vi "多点监测上位机-服务器版.vi"() -> ()   [LabVIEW 2013]
uses:
  <vilib>/Utility/miscctls.llb/LVRowAndColumnTypeDef.ctl
  <vilib>/Utility/miscctls.llb/LVRowAndColumnUnsignedTypeDef.ctl
  <vilib>/Platform/TimedLoop/XDataNode/timing_clust.ctl
  <vilib>/Platform/TimedLoop/XDataNode/nitl_modes.ctl
  <vilib>/Platform/TimedLoop/XDataNode/wakeup.ctl
  <vilib>/Utility/xml.llb/Read From XML File(string).vi
  <vilib>/sound2/lvsound2.llb/Sound File Info (path).vi
  <vilib>/sound2/lvsound2.llb/Sound File Read Open.vi
  <vilib>/sound2/lvsound2.llb/Sound File Read (DBL).vi
  <vilib>/Utility/file.llb/Read From Spreadsheet File (string).vi
  <vilib>/Utility/xml.llb/Write to XML File(string).vi
  <vilib>/Utility/file.llb/Write To Spreadsheet File (string).vi
  <vilib>/Utility/inputDevices.llb/closeMouse.vi
  <vilib>/Utility/inputDevices.llb/mouseAcquire.vi
  <vilib>/Platform/TimedLoop/XDataNode/XDataNode.xnode
  <vilib>/Platform/TimedLoop/XDataNode/XDNodeRunTimeDep.lvlib
panel:
  out "监-停止信号":refnum<vi>
  out "监测数量限值":cluster{"min":i32, "max":i32}
  in  "报警列表提示":string[](array[string])=["选行技巧：按住 ctl 可离散选择，按住 shift 可范围选择，ctl+A 选择全部行", "右键菜单：多选后 某些项可批量操作", "双击“状态”列：启用或禁用设备（某些版本中禁用此功能）", "双击“设备信息”列：修改设备信息", "双击“一级限值”列：修改报警限值", "双击“网络地址”列：删除设备", "双击“空白行”：添加设备"]
  in  "设备列表提示":string[](array[string])=["选行技巧：按住 ctl 可离散选择，按住 shift 可范围选择，ctl+A 选择全部行", "右键菜单：多选后 某些项可批量操作", "双击“状态”列：启用或禁用设备（某些版本中禁用此功能）", "双击“设备信息”列：修改设备信息", "双击“一级限值”列：修改报警限值", "双击“网络地址”列：删除设备", "双击“空白行”：添加设备"]
  in  "停止信号":enum16{"内部停止信号", "外部停止信号"}(ring)
  out "数组":errorcluster[](array[cluster])
  out "在线探头索引映射":i32[](array[numeric])
  out "在线探头":T1(array[cluster])
  out "连接断开-事件":refnum<user-event>
  out "新连接-事件":refnum<user-event>
  out "新纪录通知VI":refnum<vi>
  in  "新记录簇":cluster{"新记录列表行":string[], "对应缓存文件":string}[](array[cluster])
  in  "报警记录数":i32
  out "蜂鸣音效":waveform(dbl)[](array[waveform]) caption="数据"
  in  "新记录？":bool=TRUE
  in  "Right":i16
  in  "Left":i16
  out "最终事件":i32
  in  "所有探头数":i32
  out "定时循环结构名称":string="采集探头属性"
  in  "测量状态":enum16{"正常", "一级报警", "二级报警"}(ring)
  in  "通信单元-探头属性引用[]":refnum<vi>[](array[refnum])
  in  "通信分支-改动项引用[]":refnum<vi>[](array[refnum])
  in  "探头属性数组":T1(array[cluster])
  in  "菜单项-报警列表":enum16{"刷新", "预览并生成报表", "删除记录", "复制选中项至剪贴板"}(ring)=enum."预览并生成报表"
  in  "菜单项-实时列表":T2(ring)=enum."禁用"
  out "监测窗口VI":refnum<vi>
  out "报警记录缓存数据文件":string[](array[string])
  in  "状态与编辑":bool
  in  "监测模式":bool caption="方格样式"
  in  "查看报表":bool caption="方格样式"
  in  "设置":bool
  in  "通知设置":bool caption="方格样式"
  in  "帮助":bool
  out "公司LOGO与型号":bool
  out "设备列表标题":enum16{"设备管理列表"}(ring)
  out "设备列表操作提示":string
  in  "状态栏-项名[]":string[](array[string])
  in  "通信分支-VI引用[]":refnum<vi>[](array[refnum])
  in  "实时数据列表":i32[](listbox)
  out "报警列表标题":enum16{"报警记录列表"}(ring)
  out "报警列表操作提示":string
  in  "T:G,F:B":bool
  in  "回复背景色锁":bool
  in  "等待时间（毫秒）":u32=10
  in  "报警记录列表":i32[](listbox)
  in  "状态类型":enum16{"全部", "报警", "通信", "设置"}(ring)
  in  "暂停更新？":bool
  in  "状态栏":i32(listbox)
  in  "开机启动":bool
  in  "device ID":refnum<k1> caption="设备ID"
  in  "监测模式？":bool
  out "点到行列-实时列表":T3 caption="单元格位置"
  out "点到行列-报警记录":T3 caption="单元格位置"
  out "停止":bool=TRUE
  in  "清除状态":bool
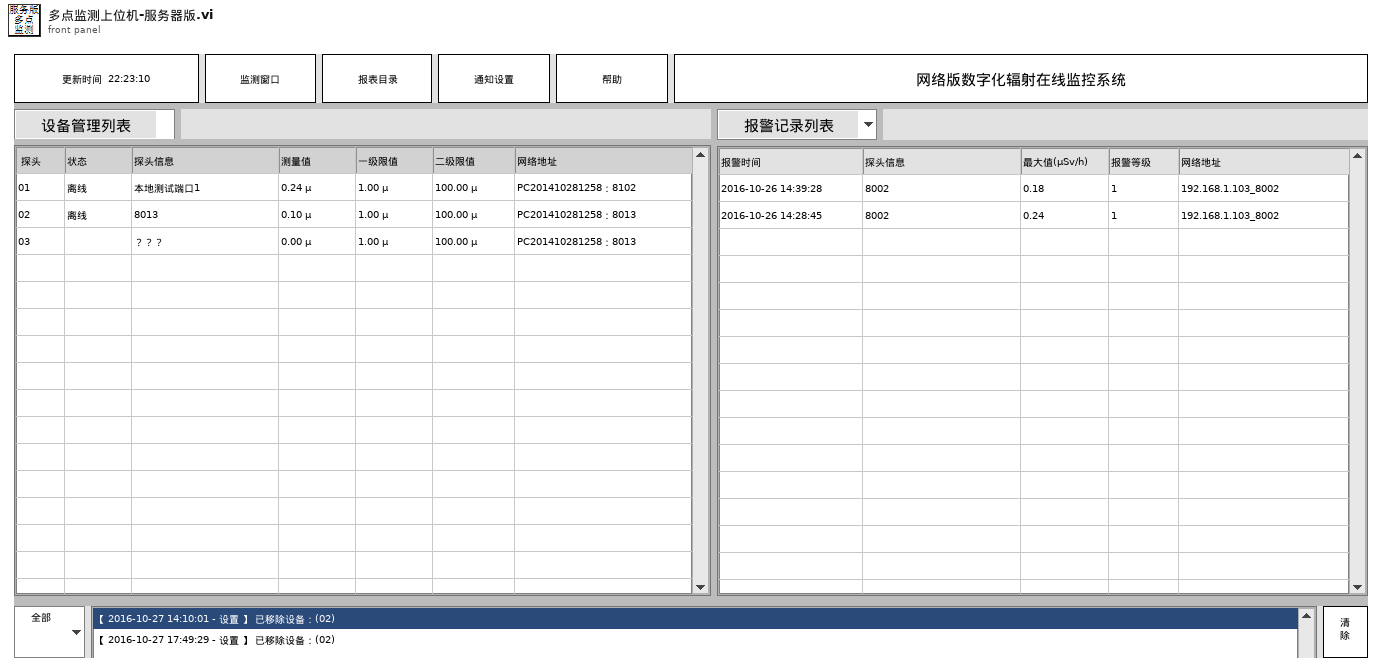
[diagram p1: front panel]
types:
  T1 = cluster{"探头地址与信息":cluster{"网络地址":cluster{"IP":string, "port":u16}, "探头信息":string}, "测量值":cluster{"时间":timestamp, "数值":dbl}, "限值":cluster{"限值1":dbl, "限值2":dbl}, "探头状态":enum16{"正常", "离线", "禁用", "一级报警", "二级报警"}}[]
  T2 = enum16{"启用", "禁用", "修改探头信息", "修改报警限值", "设备排序", "添加设备", "删除设备"}
  T3 = typedef "LVRowAndColumnTypeDef.ctl" = cluster{"Row":i32, "Column":i32}
  T4 = typedef "LVRowAndColumnUnsignedTypeDef.ctl" = cluster{"Row":u32, "Column":u32}
  T5 = enum32{"Invalid", "Standard", "Closed", "Hidden", "Minimized", "Maximized"}
  T6 = enum8{"Enabled", "Disabled", "Disabled and Grayed Out"}
  T7 = typedef "XDNodeRunTimeDep.lvlib/timing_clust.ctl" = cluster{"Expected End [f-1]":u64, "Actual End [f-1]":u64, "Finished Late? [f-1]":bool, "Expected End [i-1]":u64, "Actual End [i-1]":u64, "Finished Late? [i-1]":bool, "Expected Start [i]":u64, "Actual Start [i]":u64, "Expected Start [f]":u64, "Actual Start [f]":u64, "Source Name":string, "Structure Name":string, "Period":i64, "Deadline":i64, "Offset":i64, "Start":i64, "Priority":i32, "Timeout":i32, "Mode":T8, "Wakeup Reason":T9, "Error":errorcluster, "Source Type":string, "Secondary Source Type":string, "Global End Time":u64, "Global Start Time":u64, "Frame Duration":u64, "Iteration Duration":u64, "Assigned CPU":i32, "I/O Scan Engine Mode":u32}
  T8 = typedef "XDNodeRunTimeDep.lvlib/nitl_modes.ctl" = enum32{"No Change", "Process missed periods, maintain original phase", "Discard missed periods, maintain original phase", "Process missed periods, ignore original phase", "Discard missed periods, ignore original phase"}
  T9 = typedef "XDNodeRunTimeDep.lvlib/wakeup.ctl" = enum32{"Normal", "Aborted", "Asynchronous wakeup", "Timing source error", "Timed loop error", "Timeout"}
  T10 = cluster{"企业编号":string, "员工编号":string, "通道号":string, "密码":string, "联系人数组":cluster{"姓名":string, "手机号":string}[]}
  T11 = cluster{"连接ID":refnum<k5>, "IP地址":string, "端口":u16}
  T12 = typedef "Sound File Refnum.ctl" = refnum<file>
  T13 = typedef "LVRectTypeDef.ctl" = cluster{"Left":i16, "Top":i16, "Right":i16, "Bottom":i16}
  T14 = cluster{"探头地址与信息":cluster{"网络地址":cluster{"IP":string, "port":u16}, "探头信息":string}, "测量值":cluster{"时间":timestamp, "数值":dbl}, "限值":cluster{"限值1":dbl, "限值2":dbl}, "探头状态":enum16{"正常", "离线", "禁用", "一级报警", "二级报警"}}
  T15 = typedef "LVPoint32TypeDef.ctl" = cluster{"Horizontal":i32, "Vertical":i32}
  T16 = cluster{"button 1":bool, "button 2":bool, "button 3":bool, "button 4":bool}
  T17 = cluster{"Shift":bool, "Ctrl":bool, "Alt":bool, "Cmd":bool, "Opt":bool}
  T18 = cluster{"探头信息":string, "启用？":bool, "改动项":enum16{"未改动", "改动-探头信息", "改动-启用状态", "改动-限值"}, "限值":cluster{"限值1":dbl, "限值2":dbl}}
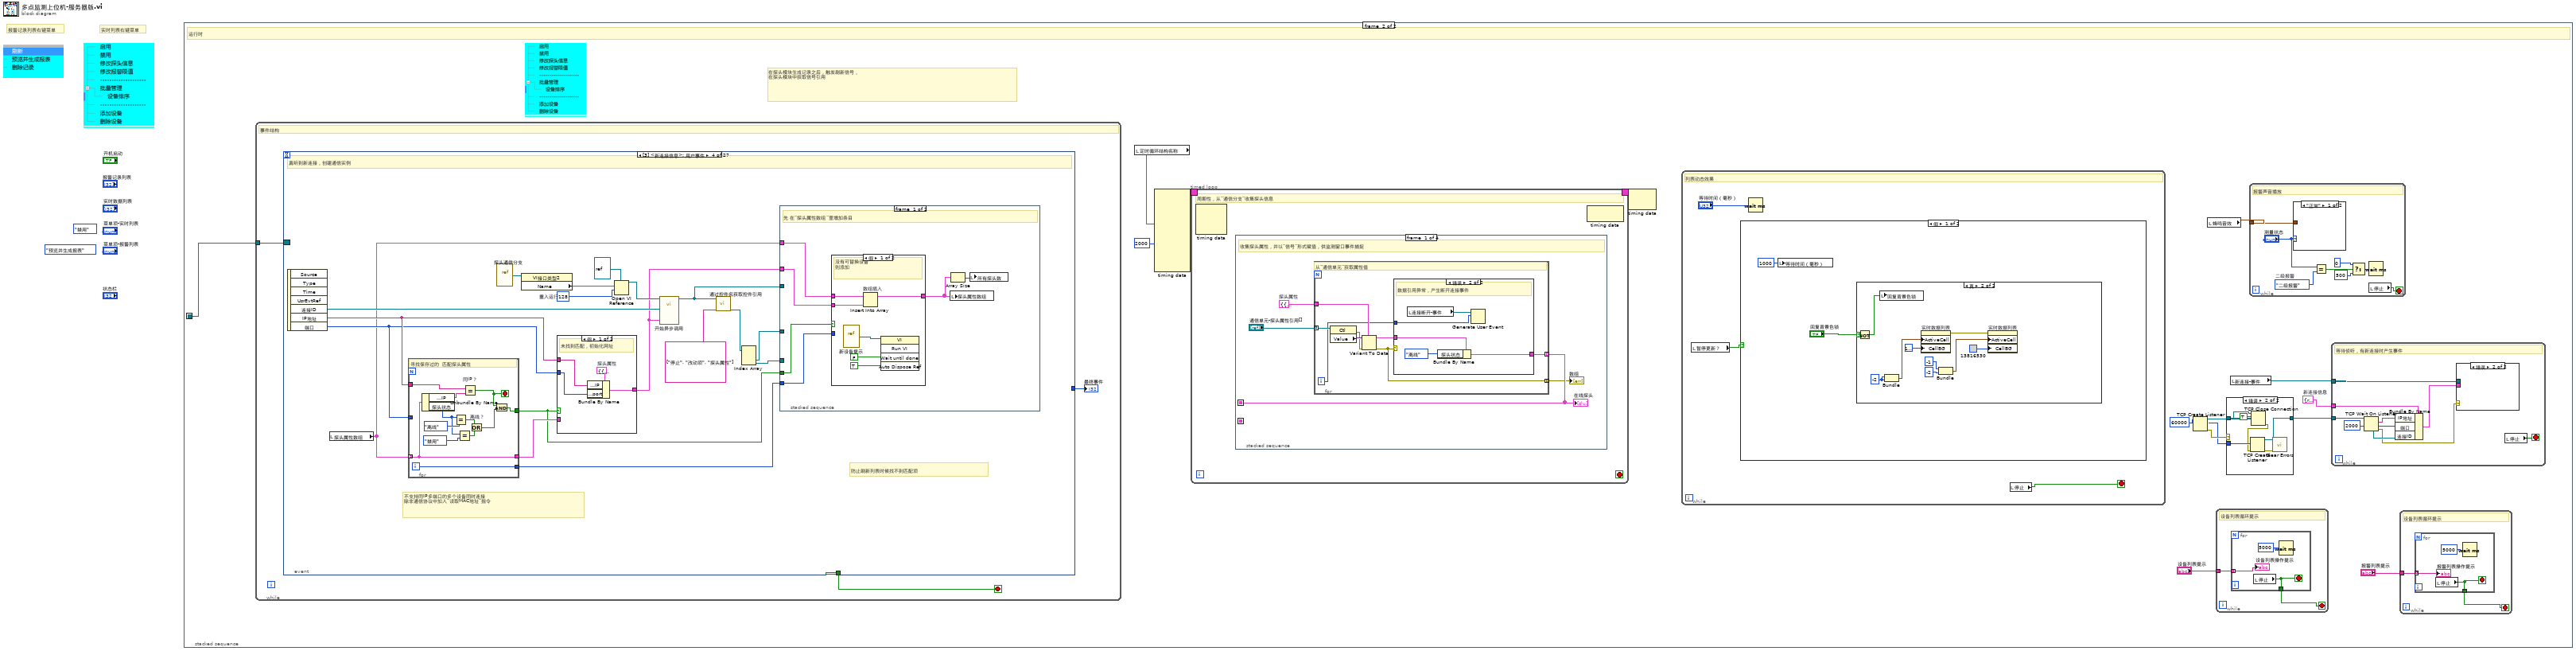
[diagram p0: block diagram]
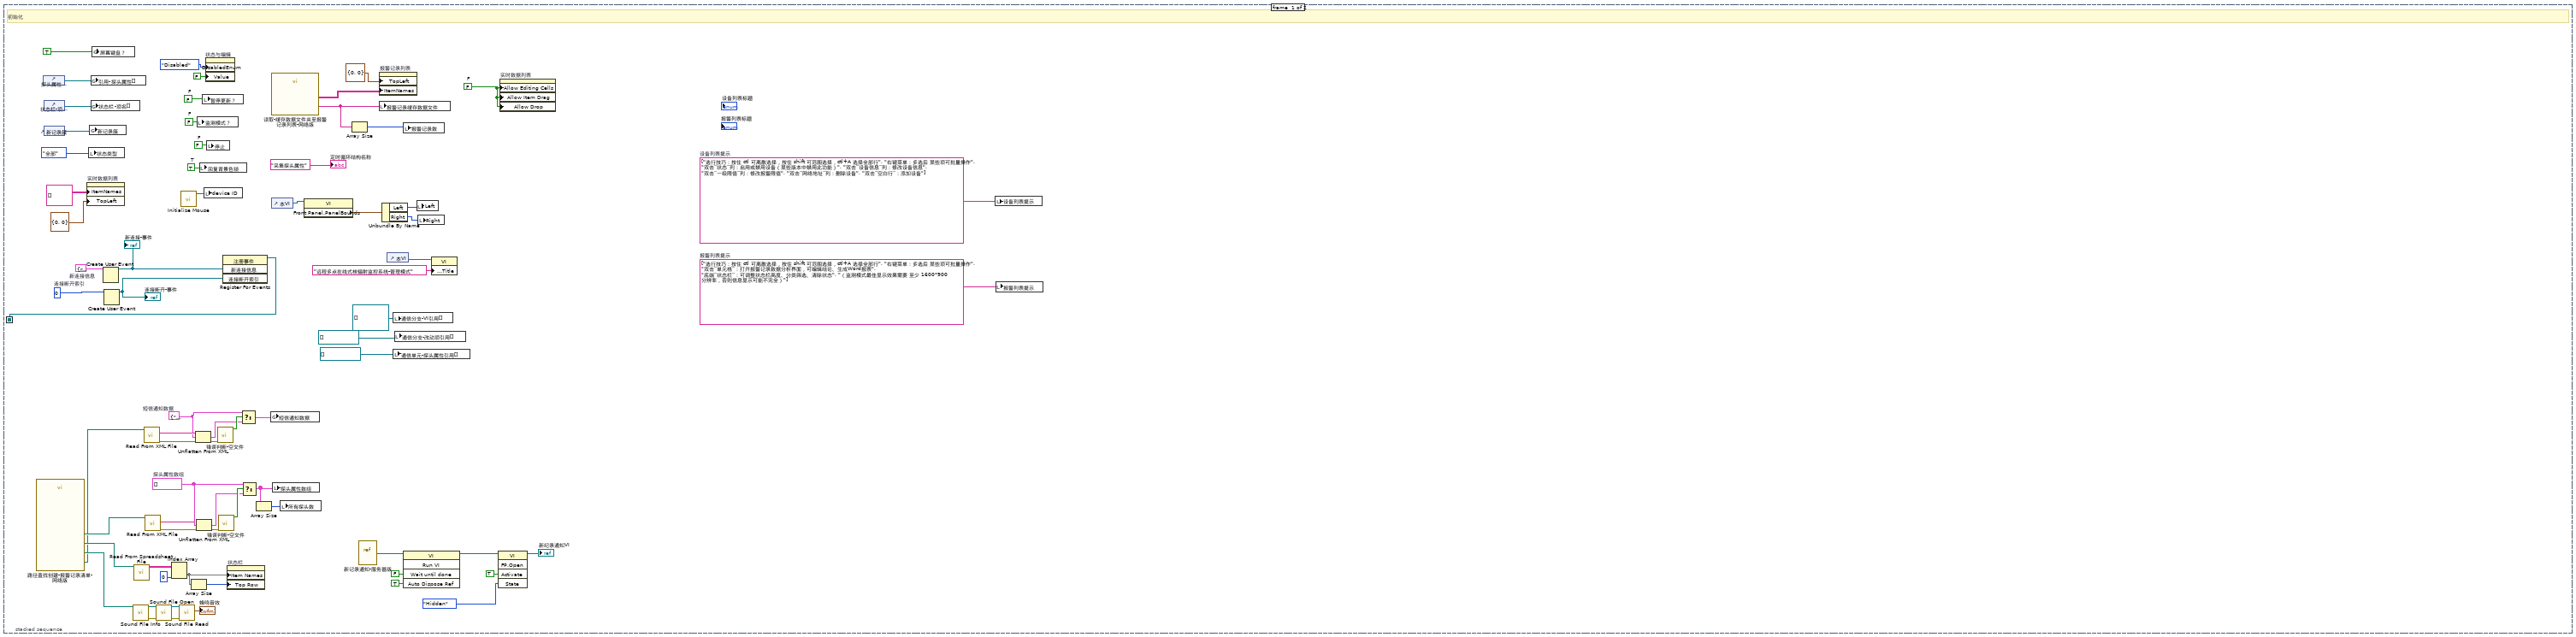
[diagram p2: hidden frame]
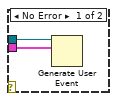
[diagram p4: hidden frame]
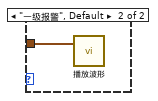
[diagram p5: hidden frame]
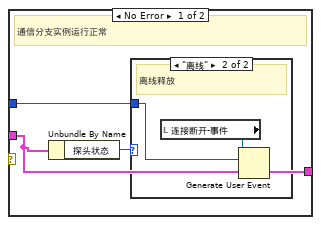
[diagram p6: hidden frame]
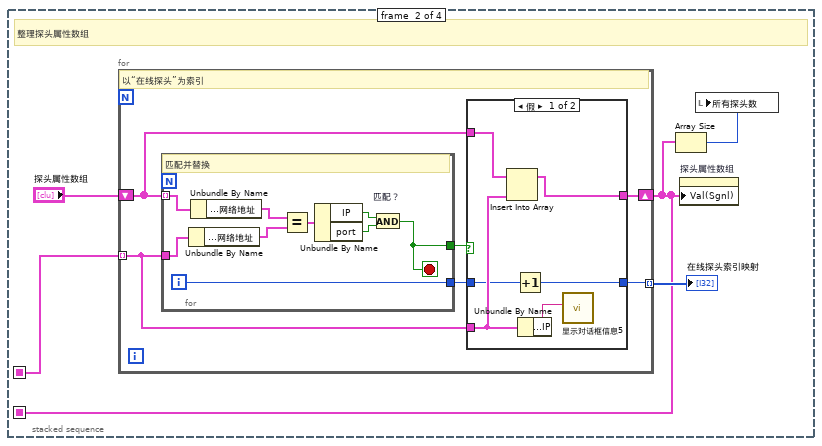
[diagram p8: hidden frame]
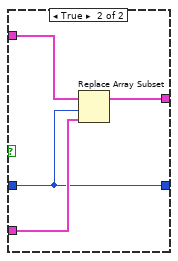
[diagram p9: hidden frame]
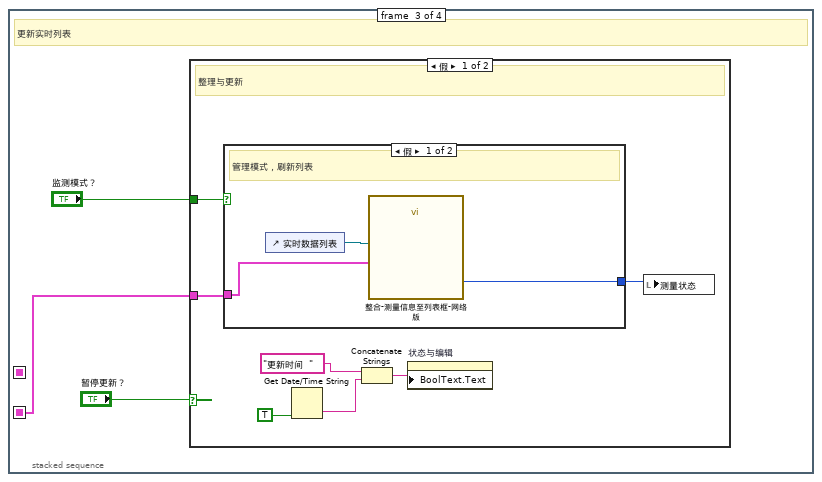
[diagram p10: hidden frame]
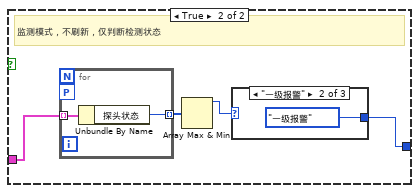
[diagram p11: hidden frame]
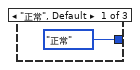
[diagram p12: hidden frame]
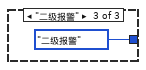
[diagram p13: hidden frame]
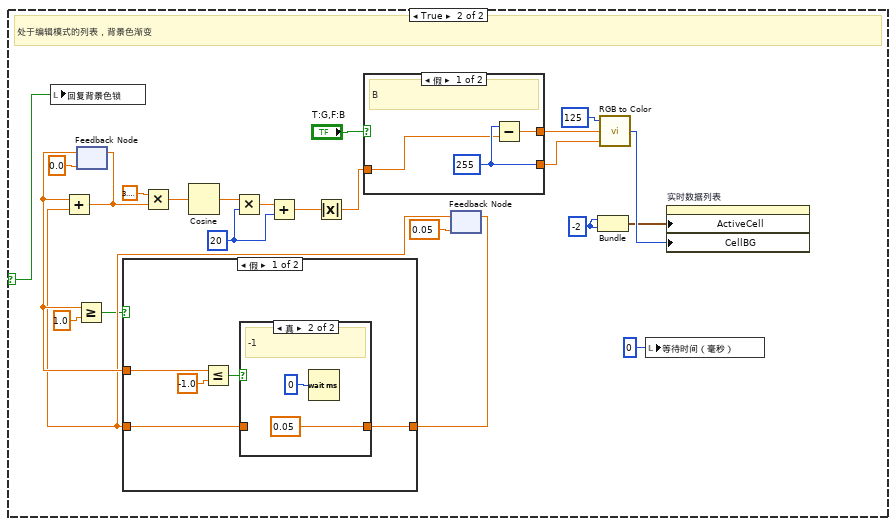
[diagram p17: hidden frame]
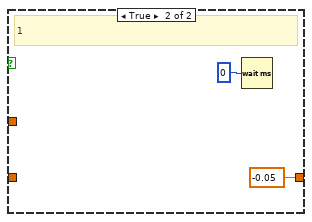
[diagram p19: hidden frame]
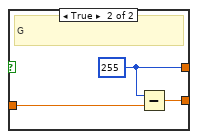
[diagram p20: hidden frame]
diagram:
  (unwired) enum16{"刷新", "预览并生成报表", "删除记录", "复制选中项至剪贴板"}."预览并生成报表" ("菜单项-报警列表")
  (unwired) T2."禁用" ("菜单项-实时列表")
  # "报警记录列表右键菜单"
  # "实时列表右键菜单"
  n1 = stacked-sequence {
    seq-local: [w24 _] -> [_ w82]
    frame #0 {
      w7 = string[] ["选行技巧：按住 ctl 可离散选择，按住 shift 可范围选择，ctl+A 选择全部行", "右键菜单：多选后 某些项可批量操作", "双击“单元格”：打开报警记录数据分析界面，可编辑结论、生成Word报表", "底端“状态栏”：可调整状态栏高度、分类筛选、清除状态", "（监测模式最佳显示效果需要 至少 1600*900 分辨率，否则信息显示可能不完全）"]  # 报警列表提示
      w6 = string[] ["选行技巧：按住 ctl 可离散选择，按住 shift 可范围选择，ctl+A 选择全部行", "右键菜单：多选后 某些项可批量操作", "双击“状态”列：启用或禁用设备（某些版本中禁用此功能）", "双击“设备信息”列：修改设备信息", "双击“一级限值”列：修改报警限值", "双击“网络地址”列：删除设备", "双击“空白行”：添加设备"]  # 设备列表提示
      w10 = T10 {"企业编号"="", "员工编号"="", "通道号"="", "密码"="", "联系人数组"=[]}  # 短信通知数据
      w22 = 0  # 连接断开索引
      w26 = T11 {"连接ID"=refnum, "IP地址"="", "端口"=0}  # 新连接信息
      w50 = TRUE  # T
      w51 = FALSE  # F
      w59 = T1 []  # 探头属性数组
      w68 = FALSE  # F
      w64 = FALSE  # F
      w71 = FALSE  # F
      # "初始化"
      n2 = call "路径查找创建-报警记录清单-网络版.vi"() -> ("探头属性配置文件"=w58:path, "状态栏信息文件"=w54:path, "蜂鸣音效文件路径"=w38:path, "短信通知配置文件"=w13:path)  [unwired: 1 in, 7 out]
      n3 = control-ref of="探头属性数组"() -> (w62:refnum<vi>)
      n4 = control-ref of="状态栏-项名[]"() -> (w70:refnum<vi>)
      n5 = control-ref of="新记录簇"() -> (w35:refnum<vi>)
      n6 = property on="实时数据列表" class="MCListbox (严格)"("ItemNames"=string[][] [] ("项名"), "TopLeft"=T4 {"Row"=0, "Column"=0} ("左上可见单元格")) -> ()  [unwired: 2 in, 2 out]
      n7 = local write "状态类型"(enum16{"全部", "报警", "通信", "设置"}."全部" ("状态类型")) -> ()
      n8 = global write "全局变量-35点监测.vi" "新记录簇"(w35) -> ()
      n9 = global write "全局变量-35点监测.vi" "引用-探头属性[]"(w62) -> ()
      n10 = global write "全局变量-35点监测.vi" "状态栏-项名[]"(w70) -> ()
      n11 = global write "全局变量-35点监测.vi" "屏幕键盘？"(TRUE ("屏幕键盘？")) -> ()
      n12 = Create User Event(user event datatype=w26) -> (user event=w25:refnum<user-event>)  [unwired: 1 in, 1 out]
      "新连接-事件" <- w25
      n13 = Create User Event(user event datatype=w22) -> (user event=w23:refnum<user-event>)  [unwired: 1 in, 1 out]
      "连接断开-事件" <- w23
      n14 = call-poly <vilib>:"Sound File Info.vi"("path"=w38) -> ("error out"=w40:errorcluster, "path out"=w41:path)  [unwired: 7 in, 2 out]
      n15 = call-poly <vilib>:"Read From Spreadsheet File.vi"("file path (dialog if empty)"=w54) -> ("all rows"=w53:string[][])  [unwired: 6 in, 4 out]
      n16 = call-poly <vilib>:"Read From XML File.vi"("XML File Path"=w13) -> ("error out"=w15:errorcluster, "XML Elements"=w12:string)  [unwired: 8 in, 1 out]
      n17 = call-poly <vilib>:"Read From XML File.vi"("XML File Path"=w58) -> ("error out"=w56:errorcluster, "XML Elements"=w55:string)  [unwired: 8 in, 1 out]
      n18 = call-poly <vilib>:"Sound File Open.vi"("error in (no error)"=w40, "path"=w41) -> ("error out"=w39:errorcluster, "sound file refnum"=w42:T12)  [unwired: 8 in]
      n19 = Index Array(array=w53, index (col)=0 ("禁用的索引 (列)")) -> (element=w19:string[])  [unwired: 1 in]
      n20 = call-poly <vilib>:"Sound File Read.vi"("error in (no error)"=w39, "sound file refnum"=w42) -> ("data"=→"蜂鸣音效":waveform(dbl)[])  [unwired: 5 in, 4 out]
      n21 = call <vilib>:"Initialize Mouse.vi"() -> ("device ID"=w69:refnum<k1>)  [unwired: 10 in, 1 out]
      n22 = Array Size(array=w19) -> (size(s)=w18:i32)
      n23 = Unflatten From XML(xml string=w12, type=w10, error in (no error)=w15) -> (value=w9:T10, error out=w14:errorcluster)
      n24 = Unflatten From XML(xml string=w55, type=w59, error in (no error)=w56) -> (value=w57:T1, error out=w60:errorcluster)
      n25 = local write "监测模式？"(w68) -> ()
      n26 = local write "回复背景色锁"(w50) -> ()
      n27 = local write "暂停更新？"(w51) -> ()
      n28 = local write "device ID"(w69) -> ()
      n29 = property on="状态与编辑" class="Bool (严格)"("DisabledEnum"=T6."Disabled" ("禁用"), "Value"=FALSE ("状态与编辑")) -> ()  [unwired: 2 in, 2 out]
      n30 = local write "停止"(w71) -> ()
      n31 = call "错误判断-空文件.vi"("错误输入"=w14) -> ("空文件？"=w11:bool)  [unwired: 9 in, 1 out]
      n32 = call "错误判断-空文件.vi"("错误输入"=w60) -> ("空文件？"=w61:bool)  [unwired: 9 in, 1 out]
      n33 = register-events(w25, w23) -> (reference out=w24:refnum<event-registration>)  [unwired: 2 in, 1 out]
      n34 = property on="状态栏" class="LstBox (严格)"("Item Names"=w19, "Top Row"=w18) -> ()  [unwired: 2 in, 2 out]
      n35 = Select(t=w10, s=w11, f=w9) -> (s? t:f=w8:T10)
      n36 = Select(t=w59, s=w61, f=w57) -> (s? t:f=w20:T1)
      n37 = Array Size(array=w20) -> (size(s)=w21:i32)
      n38 = global write "全局变量-35点监测.vi" "短信通知数据"(w8) -> ()
      n39 = call "读取-缓存数据文件夹至报警记录列表-网络版.vi"() -> ("文件名"=w37:string[], "报警记录列表"=w45:string[][])  [unwired: 8 in, 2 out]
      n40 = control-ref of="本VI"() -> (w49:refnum<vi>)
      n41 = local write "探头属性数组"(w20) -> ()
      n42 = local write "所有探头数"(w21) -> ()
      n43 = property class="VI"(reference=w49) -> ("Front Panel.PanelBounds"=w48:T13)  [unwired: 1 in, 2 out]
      n44 = Array Size(array=w37) -> (size(s)=w36:i32)
      n45 = vi-ref "新记录通知-服务器版.vi"() -> (w34:refnum<vi>)
      n46 = local write "报警记录缓存数据文件"(w37) -> ()
      n47 = property on="报警记录列表" class="MCListbox (严格)"("TopLeft"=T4 {"Row"=0, "Column"=0} ("左上可见单元格"), "ItemNames"=w45) -> ()  [unwired: 2 in, 2 out]
      n48 = Unbundle By Name(w48) -> ("Left"=w47:i16, "Right"=w46:i16)
      n49 = control-ref of="本VI"() -> (w17:refnum<vi>)
      n50 = local write "通信单元-探头属性引用[]"(refnum<vi>[] [] ("通信单元-探头属性引用[]")) -> ()
      n51 = local write "通信分支-VI引用[]"(refnum<vi>[] [] ("通信分支-VI引用[]")) -> ()
      n52 = local write "通信分支-改动项引用[]"(refnum<vi>[] [] ("通信分支-改动项引用[]")) -> ()
      n53 = local write "报警记录数"(w36) -> ()
      n54 = invoke class="VI" method="Run VI"(reference=w34, "Wait until done"=FALSE ("结束前等待"), "Auto Dispose Ref"=TRUE ("自动销毁引用")) -> (reference out=w31:refnum<vi>)  [unwired: 2 in, 4 out]
      n55 = local write "Left"(w47) -> ()
      n56 = local write "Right"(w46) -> ()
      n57 = property class="VI"(reference=w17, "Front Panel.Title"="远程多点在线式核辐射监控系统-管理模式" ("前面板窗口:标题")) -> ()  [unwired: 1 in, 2 out]
      n58 = invoke class="VI" method="FP.Open"(reference=w31, "Activate"=TRUE ("激活？"), "State"=T5."Hidden" ("状态")) -> (reference out=→"新纪录通知VI":refnum<vi>)  [unwired: 2 in, 4 out]
      n59 = property on="实时数据列表" class="多列列表框 (严格)"("Allow Editing Cells"=w64, "Allow Item Drag"=w64, "Allow Drop"=w64) -> ()  [unwired: 2 in, 2 out]
      n60 = local write "设备列表提示"(w6) -> ()
      n61 = local write "报警列表提示"(w7) -> ()
      "定时循环结构名称" <- "采集探头属性"
    }
    frame #1 {
      w80 = T11 {"连接ID"=refnum, "IP地址"="", "端口"=0}  # 新连接信息
      # "在探头模块生成记录之后，触发刷新信号，\n在探头模块中获取信号引用"
      # "运行时"
      n62 = while {
        tunnel: w82 -> [w261]
        stop <- w263 stop-if-true
        # "事件结构"
        n63 = event shown="[3] <新连接信息>: 用户事件" {
          selector: w261 -> [_ _ _ _ _ _ _ _ _ _ _ _ _ _ _ _ _ _ _ _ _ _ _ _ _ _ _]
          dyn-events: _ -> [_ _ _ _ _ _ _ _ _ _ _ _ _ _ _ _ _ _ _ _ _ _ _ _ _ _ _]
          timeout: _ -> [_ _ _ _ _ _ _ _ _ _ _ _ _ _ _ _ _ _ _ _ _ _ _ _ _ _ _]
          tunnel: [_ w267 _ _ _ _ _ _ _ _ _ _ _ _ _ _ _ _ _ _ _ _ _ _ _ _ _] -> w263
          tunnel: [0 1 _ _ _ 2 3 4 5 6 7 _ 8 9 10 _ _ _ _ _ _ 17 _ _ _ _ _] -> w262
          event Timeout {
            # "超时刷新历史记录"
            n64 = event-data() -> ()  [unwired: 1 in, 3 out]
          }
          event "停止信号": Value Change {
            # "触发停止，关闭通信单元，关闭TCP连接"
            n65 = event-data() -> ("NewVal"=w265:enum16{"内部停止信号", "外部停止信号"})  [unwired: 1 in, 5 out]
            n66 = case shown="\"内部停止信号\", 默认" w265 {
              tunnel: [w268 w269] -> w267
              frame "内部停止信号", Default {
                # "内部停止信号，有弹窗"
                n67 = call "显示对话框信息3"() -> ("确定"=w268:bool)  [unwired: 10 in, 1 out]
              }
              frame "外部停止信号" {
                w269 = TRUE  # T
                # "外部停止信号，不弹窗"
              }
            }
            "停止" <- w267
            n68 = case shown="真" w267 {
              frame False {
                # "取消停止"
              }
              frame True {
                # "关闭所有通信单元VI，关闭所有TCP连接，保存配置至文件"
                n69 = stacked-sequence {
                  frame #0 {
                    w273 = TRUE  # T
                    # "保存“探头属性”和“状态栏信息”到文件，关闭鼠标引用"
                    n70 = local read "探头属性数组"() -> (w271:T1)
                    n71 = call "路径查找创建-报警记录清单-网络版.vi"() -> ("探头属性配置文件"=w277:path, "状态栏信息文件"=w275:path)  [unwired: 1 in, 9 out]
                    n72 = local read "device ID"() -> (w272:refnum<k1>)
                    n73 = call-poly <vilib>:"Close Input Device.vi"("device ID"=w272) -> ()  [unwired: 9 in, 1 out]
                    n74 = property on="状态栏" class="LstBox (严格)"() -> ("Item Names"=w274:string[])  [unwired: 2 in, 2 out]
                    n75 = for {
                      tunnel: w271 -> [w279] mode=indexing
                      tunnel: [w278] -> w270 mode=indexing
                      # "关闭时将所有探头状态置为离线"
                      n76 = in-place {
                        n77 = in-place-cluster #1(w279) -> ()  [unwired: 1 out]
                        n78 = in-place-cluster #1("探头状态"=enum16{"正常", "离线", "禁用", "一级报警", "二级报警"}."离线") -> (w278:T14)
                      }
                    }
                    n79 = call-poly <vilib>:"Write To Spreadsheet File.vi"("transpose? (no:F)"=w273, "1D data"=w274, "file path (dialog if empty)"=w275) -> ()  [unwired: 5 in, 1 out]
                    n80 = Flatten To XML(anything=w270) -> (xml string=w276:string)
                    n81 = call-poly <vilib>:"Write to XML File.vi"("XML Input"=w276, "XML File Path"=w277) -> ()  [unwired: 7 in, 3 out]
                  }
                  frame #1 {
                    # "关闭所有通信单元VI"
                    n82 = local read "通信分支-VI引用[]"() -> (w286:refnum<vi>[])
                    n83 = local read "新纪录通知VI"() -> (w285:refnum<vi>)
                    n84 = invoke class="VI" method="Abort VI"(reference=w285) -> (reference out=w284:refnum<vi>, error out=w283:errorcluster)  [unwired: 2 in, 1 out]
                    n85 = for "For循环" {
                      tunnel: w286 -> [w288] mode=indexing
                      # "中止VI"
                      n86 = invoke class="VI (严格)" method="Abort VI"(reference=w288) -> (error out=w287:errorcluster)  [unwired: 2 in, 2 out]
                      n87 = call <vilib>:"Clear Errors.vi"("error in (no error)"=w287) -> ()  [unwired: 6 in, 1 out]
                    }
                    n88 = invoke class="VI" method="FP.Close"(reference=w284, error in=w283) -> (error out=w282:errorcluster)  [unwired: 1 in, 2 out]
                    n89 = call <vilib>:"Clear Errors.vi"("error in (no error)"=w282) -> ()  [unwired: 6 in, 1 out]
                    n90 = local read "定时循环结构名称"() -> (w281:string)
                    n91 = call <vilib>:"Stop Timed Structure.vi"("name"=w281) -> ()  [unwired: 10 in, 1 out]
                  }
                  frame #2 {
                    # "关闭前面板"
                    n92 = control-ref of="本VI"() -> (w290:refnum<vi>)
                    n93 = invoke class="VI" method="FP.Close"(reference=w290) -> (error out=w289:errorcluster)  [unwired: 2 in, 2 out]
                    n94 = call <vilib>:"Clear Errors.vi"("error in (no error)"=w289) -> ()  [unwired: 6 in, 1 out]
                  }
                }
              }
            }
          }
          event Panel Close? {
            n95 = event-data() -> ()  [unwired: 1 in, 4 out]
            n96 = property on="停止信号" class="Enum (严格)"("Val(Sgnl)"=enum16{"内部停止信号", "外部停止信号"}."内部停止信号" ("值(信号)")) -> ()  [unwired: 2 in, 2 out]
            n97 = event-data("Discard?"=TRUE ("放弃？")) -> ()  [unwired: 1 in, 1 out]
          }
          event User Event {
            w304 = 128  # 重入运行
            # "不支持同IP多端口的多个设备同时连接\n除非通信协议中加入“读取MAC地址”指令"
            # "防止刷新列表时候找不到匹配项"
            # "真听到新连接，创建通信实例"
            n98 = event-data() -> ("连接ID"=w310:refnum<k5>, "IP地址"=w309:string, "端口"=w308:u16)  [unwired: 1 in, 4 out]
            n99 = local read "探头属性数组"() -> (w296:T1)
            n100 = for {
              tunnel: w296 -> [w352] mode=indexing
              tunnel: w309 -> [w354]
              tunnel: w308 -> [_]
              tunnel: [w352] -> w307
              tunnel: [w346] -> w294
              tunnel: [w344] -> w293
              i -> [w346]
              stop <- w345 stop-if-true
              # "寻找保存过的  匹配探头属性"
              n101 = Unbundle By Name(w352) -> ("探头地址与信息.网络地址.IP"=w353:string, "探头状态"=w349:enum16{"正常", "离线", "禁用", "一级报警", "二级报警"})
              n102 = Equal?(x=w349, y=enum16{"正常", "离线", "禁用", "一级报警", "二级报警"}."离线" ("探头状态")) -> (x = y?=w350:bool)
              n103 = Equal?(x=w349, y=enum16{"正常", "离线", "禁用", "一级报警", "二级报警"}."禁用" ("探头状态")) -> (x = y?=w347:bool)
              n104 = Equal? "同IP？"(x=w354, y=w353) -> (x = y?=w345:bool)
              n105 = Or "离线？"(x=w350, y=w347) -> (x .or. y?=w343:bool)
              n106 = And(x=w345, y=w343) -> (x .and. y?=w344:bool)
            }
            n107 = vi-ref "探头通信分支.vi"() -> (w306:refnum<vi>)
            n108 = property class="VI接口类型2"(reference=w306) -> ("Name"=w305:string)  [unwired: 1 in, 2 out]
            n109 = case shown="假" w293 {
              tunnel: w307 -> [_ w342]
              tunnel: [w338 w340] -> w295
              tunnel: w309 -> [w336 _]
              tunnel: w308 -> [w337 w341]
              frame False {
                w339 = T14 {"探头地址与信息"={"网络地址"={"IP"="", "port"=0}, "探头信息"=""}, "测量值"={"时间"=timestamp(3554955153.6246996 s since 1904-01-01), "数值"=0.0}, "限值"={"限值1"=1.0, "限值2"=100.0}, "探头状态"=enum."正常"}  # 探头属性
                # "未找到匹配，初始化网址"
                n110 = Bundle By Name(cluster=w339, "探头地址与信息.网络地址.IP"=w336, "探头地址与信息.网络地址.port"=w337) -> (w338:T14)
              }
              frame True {
                # "找到匹配，替换“端口”"
                n111 = Bundle By Name(cluster=w342, "探头地址与信息.网络地址.port"=w341) -> (w340:T14)
              }
            }
            n112 = Open VI Reference(type specifier VI Refnum (for type only)=refnum<vi> refnum ("类型说明符VI引用句柄（仅用于类型）"), vi path=w305, options=w304) -> (vi reference=w302:refnum<vi>)  [unwired: 3 in, 1 out]
            n113 = call-by-ref "开始异步调用"(reference=w302, "探头属性"=w295, "连接 ID"=w310) -> (reference out=w299:refnum<vi>)  [unwired: 11 in, 1 out]
            n114 = call "通过控件名获取控件引用.vi"("控件名数组"=string[] ["停止", "改动项", "探头属性"], "VI引用"=w299) -> ("控件引用输出"=w301:refnum<vi>[])  [unwired: 7 in, 2 out]
            n115 = Index Array(array=w301) -> (element #2=w298:refnum<vi>, element #3=w297:refnum<vi>)  [unwired: 3 in, 1 out]
            n116 = stacked-sequence {
              tunnel: w299 -> [_ w334]
              tunnel: w298 -> [_ w333]
              tunnel: w297 -> [_ w330]
              tunnel: w296 -> [w316 _]
              tunnel: w295 -> [w315 _]
              tunnel: w294 -> [w314 _]
              tunnel: w293 -> [w311 _]
              frame #0 {
                # "先 在“探头属性数组”里增加条目"
                n117 = case shown="假" w311 {
                  tunnel: [w322 w323] -> w313
                  tunnel: w316 -> [w321 w326]
                  tunnel: w315 -> [w320 w324]
                  tunnel: w314 -> [_ w325]
                  frame False {
                    # "没有可替换设备\n则添加"
                    n118 = vi-ref "新设备提示.vi"() -> (w317:refnum<vi>)
                    n119 = Insert Into Array "数组插入"(array=w321, new element=w320) -> (w322:T1)  [unwired: 1 in]
                    n120 = invoke class="VI" method="Run VI"(reference=w317, "Wait until done"=FALSE ("结束前等待"), "Auto Dispose Ref"=TRUE ("自动销毁引用")) -> ()  [unwired: 2 in, 5 out]
                  }
                  frame True {
                    # "存在同 IP 的离线设备"
                    n121 = Replace Array Subset "替换数组子集"(array=w326, new element=w324, index=w325) -> (w323:T1)
                  }
                }
                n122 = local write "探头属性数组"(w313) -> ()
                n123 = Array Size(array=w313) -> (size(s)=w312:i32)
                n124 = local write "所有探头数"(w312) -> ()
              }
              frame #1 {
                # "再 添加引用到数组，不需要按顺序"
                n125 = local read "通信单元-探头属性引用[]"() -> (w329:refnum<vi>[])
                n126 = Insert Into Array(array="通信分支-改动项引用[]", new element=w333) -> (w331:refnum<vi>[])  [unwired: 1 in]
                n127 = Insert Into Array(array="通信分支-VI引用[]", new element=w334) -> (w327:refnum<vi>[])  [unwired: 1 in]
                n128 = Insert Into Array(array=w329, new element=w330) -> (w328:refnum<vi>[])  [unwired: 1 in]
                n129 = local write "通信分支-VI引用[]"(w327) -> ()
                n130 = local write "通信分支-改动项引用[]"(w331) -> ()
                n131 = local write "通信单元-探头属性引用[]"(w328) -> ()
              }
            }
          }
          event User Event {
            # "删除相关数组中的引用元素"
            n132 = event-data() -> ("连接断开索引"=w355:i32)  [unwired: 1 in, 4 out]
            n133 = local read "通信单元-探头属性引用[]"() -> (w363:refnum<vi>[])
            n134 = local read "通信分支-改动项引用[]"() -> (w364:refnum<vi>[])
            n135 = local read "通信分支-VI引用[]"() -> (w365:refnum<vi>[])
            n136 = Delete From Array(array=w365, index=w355) -> (deleted portion=w359:refnum<vi>, array with subset deleted=w362:refnum<vi>[])  [unwired: 1 in]
            n137 = Delete From Array(array=w364, index=w355) -> (array with subset deleted=w361:refnum<vi>[])  [unwired: 1 in, 1 out]
            n138 = Delete From Array(array=w363, index=w355) -> (array with subset deleted=w360:refnum<vi>[])  [unwired: 1 in, 1 out]
            n139 = invoke class="VI (严格)" method="Abort VI"(reference=w359) -> (reference out=w358:refnum<vi>, error out=w357:errorcluster)  [unwired: 2 in, 1 out]
            n140 = Close Reference(reference=w358, error in (no error)=w357) -> (error out=w356:errorcluster)
            n141 = call <vilib>:"Clear Errors.vi"("error in (no error)"=w356) -> ()  [unwired: 6 in, 1 out]
            n142 = local write "通信单元-探头属性引用[]"(w360) -> ()
            n143 = local write "通信分支-VI引用[]"(w362) -> ()
            n144 = local write "通信分支-改动项引用[]"(w361) -> ()
          }
          event "实时数据列表", "报警记录列表": Mouse Down {
            # "使  右击行  列表能够获取焦点"
            n145 = event-data() -> ("CtlRef"=w371:refnum<vi>, "Coords"=w373:T15)  [unwired: 1 in, 7 out]
            n146 = property class="MCListbox (严格)"(reference=w371) -> ("Label.Text"=w370:string)  [unwired: 1 in, 2 out]
            n147 = call-poly <vilib>:"Acquire Input Data.vi"("device ID"="device ID") -> ("button info"=w375:T16)  [unwired: 15 in, 3 out]
            n148 = invoke class="多列列表框 (严格)" method="Point To Row Column"(reference=w371, "Point"=w373) -> ("CellPosition"=w372:T3)  [unwired: 5 in, 6 out]
            "点到行列-实时列表" <- w372
            n149 = property on="实时数据列表" class="MCListbox (严格)"() -> ("Label.Text"=w369:string)  [unwired: 2 in, 2 out]
            n150 = Unbundle By Name "btn_2"(w375) -> ("button 2"=w374:bool)
            n151 = Equal?(x=w370, y=w369) -> (x = y?=w368:bool)
            n152 = case shown="真" w374 {
              tunnel: w371 -> [_ w391]
              tunnel: w372 -> [_ w389]
              tunnel: w368 -> [_ w379]
              frame False {
                # "不是右键"
              }
              frame True {
                w384 = TRUE  # T
                w392 = TRUE  # T
                # "右键"
                n153 = property class="多列列表框 (严格)" props=["ContentRectPosTop", "Value"](reference=w391) -> ("Value"=w388:i32[])  [unwired: 1 in, 3 out]
                n154 = Unbundle By Name(w389) -> ("Row"=w382:i32)
                n155 = Increment(x=w382) -> (x+1=w381:i32)
                n156 = Build Array(w382) -> (w390:i32[])
                n157 = Select(t="所有探头数", s=w379, f="报警记录数") -> (s? t:f=w377:i32)
                n158 = Less Or Equal? "点在有效信息行内？"(x=w381, y=w377) -> (x <= y?=w380:bool)
                n159 = for "For循环" {
                  tunnel: w388 -> [w409] mode=indexing
                  shift-right: [w406] -> w386
                  shift-left: w392 -> [w407]
                  tunnel: w382 -> [w404]
                  tunnel: w380 -> [w403]
                  stop <- w406 continue-if-true
                  # "在选中项之外？"
                  n160 = Not Equal?(x=w409, y=w404) -> (x != y?=w408:bool)
                  n161 = Greater Or Equal To 0?(x=w404) -> (x >= 0?=w405:bool)
                  n162 = Compound Arithmetic op=AND(w408, w407, w405, w403) -> (w406:bool)
                }
                n163 = Empty Array? "空数组？"(array=w388) -> (empty?=w387:bool)
                n164 = Select(t=w384, s=w387, f=w386) -> (s? t:f=w385:bool)
                n165 = And(x=w385, y=w380) -> (x .and. y?=w383:bool)
                n166 = case shown="假" w383 {
                  tunnel: w390 -> [_ w400]
                  tunnel: w379 -> [w393 w399]
                  tunnel: w380 -> [w394 _]
                  frame False {
                    # "在选中项之中，不赋值"
                    n167 = case shown="假" w394 {
                      tunnel: w393 -> [w395 _]
                      frame False {
                        # "点在不可选行，清空"
                        n168 = case shown="假" w395 {
                          tunnel: i32[] [] ("实时数据列表") -> [w397 w398]
                          frame False {
                            # "报警记录表"
                            n169 = local write "报警记录列表"(w397) -> ()
                          }
                          frame True {
                            # "实时表"
                            n170 = local write "实时数据列表"(w398) -> ()
                          }
                        }
                      }
                      frame True {
                        # "点在可选行，不赋值"
                      }
                    }
                  }
                  frame True {
                    # "在选中项之外，赋值"
                    n171 = case shown="假" w399 {
                      tunnel: w400 -> [w401 w402]
                      frame False {
                        n172 = local write "报警记录列表"(w401) -> ()
                      }
                      frame True {
                        n173 = local write "实时数据列表"(w402) -> ()
                      }
                    }
                  }
                }
              }
            }
          }
          event "监测模式": Value Change {
            # "切换到 方格 样式 界面"
            n174 = event-data() -> ()  [unwired: 1 in, 6 out]
            n175 = stacked-sequence {
              seq-local: [w413 _] -> [_ w421]
              seq-local: [w412 _] -> [_ w420]
              frame #0 {
                # "判断是否有未命名的设备"
                n176 = local read "探头属性数组"() -> (w415:T1)
                n177 = for {
                  tunnel: w415 -> [w419] mode=indexing
                  tunnel: [w416] -> w412 mode=indexing if=w417
                  workers-P: _ -> [_]
                  # "查找未命名设备"
                  n178 = Unbundle By Name(w419) -> ("探头地址与信息.探头信息"=w418:string, "探头地址与信息.网络地址.IP"=w416:string)
                  n179 = Empty String/Path? "空字符串/路径？"(string/path=w418) -> (empty?=w417:bool)
                }
                n180 = Array Size(array=w412) -> (size(s)=w414:i32)
                n181 = Equal To 0?(x=w414) -> (x = 0?=w413:bool)
              }
              frame #1 {
                # "切换到监测模式"
                n182 = case shown="真" w421 {
                  tunnel: w420 -> [w433 _]
                  frame False {
                    w423 = "\r"
                    w428 = "……"  # 更多设备
                    w431 = 3
                    n183 = Array Size(array=w433) -> (size(s)=w432:i32)
                    n184 = for {
                      N: w431 -> [_]
                      tunnel: w433 -> [w436] mode=indexing
                      shift-right: [w434] -> w426
                      shift-left: "" -> [w437]
                      # "列举前三个未命名设备"
                      n185 = Concatenate Strings(w437, w436, "\r") -> (w434:string)
                    }
                    n186 = Greater?(x=w432, y=w431) -> (0:w430:bool)
                    n187 = Select(t=w428, s=w430, f="") -> (s? t:f=w425:string)
                    n188 = Concatenate Strings("存在待命名的设备" ("字符串"), w423, w426, w425, w423) -> (w422:string)
                    n189 = call "显示对话框信息6"("Message"=w422) -> ()  [unwired: 9 in, 2 out]
                  }
                  frame True {
                    n190 = local read "所有探头数"() -> (w440:i32)
                    n191 = local read "暂停更新？"() -> (w443:bool)
                    n192 = Equal To 0? "没有探头"(x=w440) -> (x = 0?=w441:bool)
                    n193 = Or(x=w441, y=w443) -> (x .or. y?=w442:bool)
                    n194 = Less Or Equal?(x=w440, y=32) -> (x <= y?=w438:bool)
                    n195 = case shown="真" w438 {
                      tunnel: w442 -> [_ w445]
                      tunnel: w440 -> [_ w444]
                      frame False {
                        # "超过32个探头，不能打开监测界面"
                        n196 = call "显示对话框信息4"() -> ()  [unwired: 10 in, 2 out]
                      }
                      frame True {
                        # "32个探头内可打开监测界面"
                        n197 = case shown="假" w445 {
                          tunnel: w444 -> [w448 _]
                          frame False {
                            # "正常更新列表中，表示没有未完成的设置操作"
                            n198 = case shown="29..32" w448 {
                              tunnel: [w461 w463 w465 w467 w469 w471 w473 w475 w477 w479] -> w447
                              tunnel: [cluster{"min":i32, "max":i32} {"min"=0, "max"=2} ("监测数量限值") cluster{"min":i32, "max":i32} {"min"=3, "max"=4} ("监测数量限值") cluster{"min":i32, "max":i32} {"min"=5, "max"=6} ("监测数量限值") cluster{"min":i32, "max":i32} {"min"=7, "max"=8} ("监测数量限值") cluster{"min":i32, "max":i32} {"min"=9, "max"=12} ("监测数量限值") cluster{"min":i32, "max":i32} {"min"=13, "max"=16} ("监测数量限值") cluster{"min":i32, "max":i32} {"min"=17, "max"=20} ("监测数量限值") cluster{"min":i32, "max":i32} {"min"=21, "max"=24} ("监测数量限值") cluster{"min":i32, "max":i32} {"min"=25, "max"=28} ("监测数量限值") cluster{"min":i32, "max":i32} {"min"=29, "max"=32} ("监测数量限值")] -> w446
                              frame 0..2, Default {
                                n199 = vi-ref "探头窗口-2-网络版.vi"() -> (w461:refnum<vi>)
                              }
                              frame 3, 4 {
                                n200 = vi-ref "探头窗口-4-网络版.vi"() -> (w463:refnum<vi>)
                              }
                              frame 5, 6 {
                                n201 = vi-ref "探头窗口-6-网络版.vi"() -> (w465:refnum<vi>)
                              }
                              frame 7, 8 {
                                n202 = vi-ref "探头窗口-8-网络版.vi"() -> (w467:refnum<vi>)
                              }
                              frame 9..12 {
                                n203 = vi-ref "探头窗口-12-网络版.vi"() -> (w469:refnum<vi>)
                              }
                              frame 13..16 {
                                n204 = vi-ref "探头窗口-16-网络版.vi"() -> (w471:refnum<vi>)
                              }
                              frame 17..20 {
                                n205 = vi-ref "探头窗口-20-网络版.vi"() -> (w473:refnum<vi>)
                              }
                              frame 21..24 {
                                n206 = vi-ref "探头窗口-24-4列-网络版.vi"() -> (w475:refnum<vi>)
                              }
                              frame 25..28 {
                                n207 = vi-ref "探头窗口-28-4列-网络版.vi"() -> (w477:refnum<vi>)
                              }
                              frame 29..32 {
                                n208 = vi-ref "探头窗口-32-4列-网络版.vi"() -> (w479:refnum<vi>)
                              }
                            }
                            "监测数量限值" <- w446
                            n209 = invoke on="运行VI" class="VI" method="Run VI"(reference=w447, "Wait until done"=FALSE ("结束前等待"), "Auto Dispose Ref"=TRUE ("自动销毁引用")) -> (reference out=w453:refnum<vi>, error out=w454:errorcluster)  [unwired: 2 in, 3 out]
                            n210 = disable-structure shown="禁用" {
                              disable-tunnel: w454 -> [w488 w493]
                              disable-tunnel: w453 -> [w486 w494]
                              disable-tunnel: [w481 w493] -> w450
                              disable-tunnel: [w480 w494] -> w449
                              frame Disabled {
                                # "没有顶层框架时候，启用"
                                n211 = control-ref of="本VI"() -> (w484:refnum<vi>)
                                n212 = invoke on="打开前面板" class="VI" method="FP.Open"(reference=w486, error in=w488, "Activate"=TRUE ("激活？"), "State"=T5."Maximized" ("状态")) -> (reference out=w480:refnum<vi>, error out=w483:errorcluster)  [unwired: 1 in, 3 out]
                                n213 = disable-structure shown="启用" {
                                disable-tunnel: w484 -> [w492 _]
                                disable-tunnel: w483 -> [w491 _]
                                disable-tunnel: T5."Hidden" ("前面板窗口:状态") -> [w490 _]
                                disable-tunnel: [w489 _] -> w481
                                frame Enabled {
                                n214 = property class="VI"(reference=w492, error in=w491, "FP.State"=w490) -> (error out=w489:errorcluster)  [unwired: 1 out]
                                }
                                frame Disabled {
                                }
                                }
                              }
                              frame Enabled {
                              }
                            }
                            n215 = stacked-sequence {
                              tunnel: w449 -> [w455 _]
                              frame #0 {
                                n216 = call "通过控件名获取控件引用.vi"("控件名数组"=string[] ["外部停止命令？"], "VI引用"=w455) -> ("控件引用输出"=w456:refnum<vi>[])  [unwired: 7 in, 2 out]
                                n217 = Index Array(array=w456) -> (element=→"监-停止信号":refnum<vi>)  [unwired: 1 in]
                                "监测窗口VI" <- w455
                              }
                              frame #1 {
                                w459 = TRUE  # Y
                                n218 = property on="监测模式？" class="Bool (严格)"("Val(Sgnl)"=w459) -> ()  [unwired: 2 in, 2 out]
                              }
                            }
                            n219 = call <vilib>:"Clear Errors.vi"("error in (no error)"=w450) -> ()  [unwired: 6 in, 1 out]
                          }
                          frame True {
                            # "存在未完成的设置操作，弹窗提示"
                            n220 = call "显示对话框信息2"() -> ()  [unwired: 10 in, 2 out]
                          }
                        }
                      }
                    }
                  }
                }
              }
            }
            n221 = local write "监测模式"(FALSE ("监测模式")) -> ()
          }
          event "查看报表": Value Change {
            # "打开文件路径"
            n222 = event-data() -> ()  [unwired: 1 in, 6 out]
            n223 = call "路径查找创建-报警记录清单-网络版.vi"() -> ("报表文件夹"=w496:path)  [unwired: 1 in, 10 out]
            n224 = call "cmd打开文件夹.vi"("文件路径"=w496) -> ()  [unwired: 10 in, 1 out]
          }
          event "帮助": Value Change {
            n225 = event-data() -> ()  [unwired: 1 in, 6 out]
            n226 = call "路径查找创建-报警记录清单-网络版.vi"() -> ("Server 版帮助文档路径"=w497:path)  [unwired: 1 in, 10 out]
            n227 = call "cmd打开文件.vi"("文件路径"=w497) -> ()  [unwired: 10 in, 1 out]
          }
          event "公司LOGO与型号": Mouse Up {
            n228 = event-data() -> ("Mods.Double Click"=w500:bool)  [unwired: 1 in, 7 out]
            n229 = case shown="假" w500 {
              frame False {
              }
              frame True {
                # "双击打开网址"
              }
            }
          }
          event "状态栏-项名[]": Value Change {
            # "在其他VI里改变值，在此处处理"
            n230 = event-data() -> ()  [unwired: 1 in, 6 out]
            n231 = local read "状态类型"() -> (w505:enum16{"全部", "报警", "通信", "设置"})
            n232 = Array Size(array="状态栏-项名[]") -> (size(s)=w508:i32)
            n233 = Decrement(x=w508) -> (x-1=w509:i32)
            n234 = Index Array "获取新增项"(array="状态栏-项名[]", index=w509) -> (element=w504:string)
            n235 = Equal To 0?(x=w505) -> (x = 0?=w506:bool)
            n236 = case shown="假" w506 {
              tunnel: w505 -> [w525 _]
              tunnel: w504 -> [w523 _]
              tunnel: [w520 w526] -> w502
              frame False {
                # "按关键词过滤"
                n237 = property on="状态类型" class="Enum (严格)"() -> ("Strings []"=w519:string[])  [unwired: 2 in, 2 out]
                n238 = Index Array "当前关键词"(array=w519, index=w525) -> (element=w522:string)
                n239 = Match Pattern(string=w523, regular expression=w522, offset (0)=20 ("偏移量(0)")) -> (offset past match=w521:i32)  [unwired: 3 out]
                n240 = Greater Or Equal To 0?(x=w521) -> (x >= 0?=w520:bool)
              }
              frame True {
                w526 = TRUE  # T
                # "显示全部"
              }
            }
            n241 = control-ref of="状态栏"() -> (w503:refnum<vi>)
            n242 = case shown="真" w502 {
              tunnel: w503 -> [_ w518]
              tunnel: w504 -> [_ w514]
              frame False {
                # "未匹配，不添加"
              }
              frame True {
                # "添加，并置为左上可见"
                n243 = call-poly "多态-列表插入项名.vi"("项名"=w514, "限定行数(500)"=u32 500, "LstBox引用句柄"=w518) -> ("引用输出"=w517:refnum<vi>)  [unwired: 8 in]
                n244 = property class="LstBox"(reference=w517) -> (reference out=w516:refnum<vi>, error out=w515:errorcluster, "Item Names"=w513:string[])  [unwired: 1 in]
                n245 = Array Size(array=w513) -> (size(s)=w512:i32)
                n246 = Decrement(x=w512) -> (x-1=w511:i32)
                n247 = property class="LstBox"(reference=w516, error in=w515, "Top Row"=w511) -> ()  [unwired: 2 out]
              }
            }
          }
          event "通知设置": Value Change {
            # "打开通知设置窗口"
            n248 = event-data() -> ()  [unwired: 1 in, 6 out]
            n249 = vi-ref "短信通知设置.vi"() -> (w530:refnum<vi>)
            n250 = invoke class="VI" method="Run VI"(reference=w530, "Wait until done"=FALSE ("结束前等待"), "Auto Dispose Ref"=TRUE ("自动销毁引用")) -> (error out=w527:errorcluster)  [unwired: 2 in, 4 out]
            n251 = call <vilib>:"Clear Errors.vi"("error in (no error)"=w527) -> ()  [unwired: 6 in, 1 out]
          }
          event "状态类型": Value Change {
            n252 = event-data() -> ()  [unwired: 1 in, 6 out]
            n253 = local read "状态栏-项名[]"() -> (w539:string[])
            n254 = Equal To 0?(x="状态类型") -> (x = 0?=w541:bool)
            n255 = case shown="假" w541 {
              tunnel: "状态类型" -> [w549 _]
              tunnel: w539 -> [w548 w561]
              tunnel: [w546 w561] -> w533
              frame False {
                # "按关键词过滤"
                n256 = property on="状态类型" class="Enum (严格)"() -> ("Strings []"=w545:string[])  [unwired: 2 in, 2 out]
                n257 = Index Array "当前关键词"(array=w545, index=w549) -> (element=w544:string)
                n258 = Concatenate Strings(w544, " 】 ") -> (w542:string)
                n259 = for "For循环" {
                  tunnel: w548 -> [w551] mode=indexing
                  tunnel: w542 -> [w554]
                  shift-right: [w550] -> w546
                  shift-left: string[] [] ("项名") -> [w552]
                  # "过滤关键词"
                  n260 = Match Pattern(string=w551, regular expression=w554, offset (0)=20 ("偏移量(0)")) -> (offset past match=w556:i32)  [unwired: 3 out]
                  n261 = Greater Or Equal To 0?(x=w556) -> (x >= 0?=w553:bool)
                  n262 = case shown="真" w553 {
                    tunnel: w552 -> [w557 w560]
                    tunnel: w551 -> [_ w559]
                    tunnel: [w557 w558] -> w550
                    frame False {
                      # "不匹配"
                    }
                    frame True {
                      # "匹配"
                      n263 = Insert Into Array(array=w560, new element=w559) -> (w558:string[])  [unwired: 1 in]
                    }
                  }
                }
              }
              frame True {
                # "显示全部"
              }
            }
            n264 = Array Size(array=w533) -> (size(s)=w534:i32)
            n265 = Decrement(x=w534) -> (x-1=w536:i32)
            n266 = control-ref of="状态栏"() -> (w532:refnum<vi>)
            n267 = Less Than 0?(x=w536) -> (x < 0?=w535:bool)
            n268 = Select(t=0, s=w535, f=w536) -> (s? t:f=w538:i32)
            n269 = property class="LstBox (严格)"(reference=w532, "Item Names"=w533, "Top Row"=w538) -> ()  [unwired: 1 in, 2 out]
          }
          event "清除状态": Value Change {
            n270 = event-data() -> ()  [unwired: 1 in, 6 out]
            n271 = control-ref of="状态栏"() -> (w567:refnum<vi>)
            n272 = property class="LstBox (严格)"(reference=w567, "Item Names"=string[] [] ("项名")) -> ()  [unwired: 1 in, 2 out]
            n273 = local read "状态栏-项名[]"() -> (w565:string[])
            n274 = local read "状态类型"() -> (w563:enum16{"全部", "报警", "通信", "设置"})
            n275 = Equal To 0?(x=w563) -> (x = 0?=w566:bool)
            n276 = case shown="假" w566 {
              tunnel: w563 -> [w574 _]
              tunnel: w565 -> [w573 _]
              tunnel: [w570 string[] [] ("项名")] -> w564
              frame False {
                # "关键词以外的，保留"
                n277 = property on="状态类型" class="Enum (严格)"() -> ("Strings []"=w569:string[])  [unwired: 2 in, 2 out]
                n278 = Index Array "当前关键词"(array=w569, index=w574) -> (element=w572:string)
                n279 = for "For循环" {
                  tunnel: w573 -> [w576] mode=indexing
                  tunnel: w572 -> [w579]
                  shift-right: [w575] -> w570
                  shift-left: string[] [] ("项名") -> [w577]
                  # "过滤关键词"
                  n280 = Match Pattern(string=w576, regular expression=w579, offset (0)=20 ("偏移量(0)")) -> (offset past match=w581:i32)  [unwired: 3 out]
                  n281 = Less Than 0? "不匹配？"(x=w581) -> (x < 0?=w578:bool)
                  n282 = case shown="假" w578 {
                    tunnel: w577 -> [w582 w585]
                    tunnel: w576 -> [_ w584]
                    tunnel: [w582 w583] -> w575
                    frame False {
                      # "匹配\n不保留"
                    }
                    frame True {
                      # "不匹配\n保留"
                      n283 = Insert Into Array(array=w585, new element=w584) -> (w583:string[])  [unwired: 1 in]
                    }
                  }
                }
              }
              frame True {
                # "全部清除"
              }
            }
            n284 = local write "状态栏-项名[]"(w564) -> ()
          }
          event "监测模式？": Value Change {
            # "从方格窗口切换回来"
            n285 = event-data() -> ()  [unwired: 1 in, 6 out]
            n286 = disable-structure shown="禁用" {
              frame Disabled {
                # "没有顶层框架时候，启用"
                n287 = control-ref of="本VI"() -> (w589:refnum<vi>)
                n288 = invoke class="VI" method="FP.Open"(reference=w589, "Activate"=TRUE ("激活？"), "State"=T5."Standard" ("状态")) -> (error out=w588:errorcluster)  [unwired: 2 in, 4 out]
                n289 = call <vilib>:"Clear Errors.vi"("error in (no error)"=w588) -> ()  [unwired: 6 in, 1 out]
              }
              frame Enabled {
              }
            }
          }
          event "实时数据列表": Double Click {
            (unwired) T2."禁用" ("菜单项-实时列表")
            w607 = enum16{"正常", "离线", "禁用", "一级报警", "二级报警"}."离线"  # 探头状态-在线
            w609 = enum16{"正常", "离线", "禁用", "一级报警", "二级报警"}."禁用"  # 探头状态-禁用
            # "使 双击 可寻找到对应的列，并触发菜单处理事件，使打开修改弹窗"
            n290 = event-data() -> ("CtlRef"=w611:refnum<vi>, "Coords"=w615:T15, "PlatMods"=w595:T17)  [unwired: 1 in, 6 out]
            n291 = property class="MCListbox (严格)"(reference=w611) -> ("Value"=w613:i32[])  [unwired: 1 in, 2 out]
            n292 = Unbundle By Name(w595) -> ("Shift"=w597:bool, "Ctrl"=w596:bool)
            n293 = local read "探头属性数组"() -> (w598:T1)
            n294 = invoke class="多列列表框 (严格)" method="Point To Row Column"(reference=w611, "Point"=w615) -> ("CellPosition"=w616:T3)  [unwired: 5 in, 6 out]
            n295 = Not Or(1:w596, 2:w597) -> (0:w593:bool)
            n296 = Unbundle By Name(w616) -> ("Row"=w601:i32, "Column"=w614:i32)
            n297 = Index Array(array=w613) -> (element=w612:i32)  [unwired: 1 in]
            n298 = Array Size(array=w598) -> (size(s)=w604:i32)
            n299 = Index Array(array=w598, index=w612) -> (element=w610:T14)
            n300 = Decrement(x=w604) -> (x-1=w592:i32)
            n301 = Unbundle By Name(w610) -> ("探头状态"=w606:enum16{"正常", "离线", "禁用", "一级报警", "二级报警"})
            n302 = In Range and Coerce(upper limit=w592, x=w601, lower limit=0 ("下限")) -> (In Range?=w602:bool)  [unwired: 1 out]
            n303 = Not Equal? "启用？"(x=w606, y=w609) -> (x != y?=w608:bool)
            n304 = Not Equal? "在线？"(x=w607, y=w606) -> (x != y?=w605:bool)
            n305 = And(x=w602, y=w593) -> (x .and. y?=w594:bool)
            n306 = case shown="真" w594 {
              tunnel: w611 -> [_ w629]
              tunnel: w614 -> [_ w628]
              tunnel: w608 -> [_ w627]
              tunnel: w605 -> [_ w626]
              tunnel: w601 -> [w621 _]
              tunnel: [w618 w625] -> w600
              tunnel: [w619 w624] -> w599
              frame False {
                # "无效行"
                n307 = Greater Than 0?(x=w621) -> (x > 0?=w620:bool)
                n308 = case shown="真" w620 {
                  tunnel: [_ w623] -> w619
                  tunnel: [_ w622] -> w618
                  frame False {
                    # "标题行，不执行"
                  }
                  frame True {
                    w622 = T2."添加设备"  # 添加设备
                    w623 = TRUE  # T
                    # "空白行，添加设备"
                  }
                }
              }
              frame True {
                # "有效行，范围内"
                n309 = case shown="1, 2, 4..6" w628 {
                  tunnel: w628 -> [_ w635]
                  tunnel: w629 -> [_ w634]
                  tunnel: w627 -> [_ w633]
                  tunnel: w626 -> [_ w632]
                  tunnel: [_ w631] -> w625
                  tunnel: [_ w630] -> w624
                  frame -1, Default {
                    # "不触发菜单事件"
                  }
                  frame 1, 2, 4..6 {
                    # "指定列内才可以触发菜单事件"
                    n310 = case shown="4, 5" w635 {
                      tunnel: [w640 w641 w643 w647] -> w631
                      tunnel: w634 -> [_ _ _ _]
                      tunnel: w633 -> [w638 _ w645 _]
                      tunnel: [w639 w642 w644 w648] -> w630
                      tunnel: w632 -> [_ _ w646 _]
                      frame 1, Default {
                        w636 = T2."启用"  # 启用
                        w637 = T2."禁用"  # 禁用
                        w639 = TRUE  # T
                        # "状态列，禁用或启用探头"
                        n311 = Select(t=w637, s=w638, f=w636) -> (s? t:f=w640:T2)
                      }
                      frame 2 {
                        w641 = T2."修改探头信息"  # 修改探头信息
                        w642 = TRUE  # T
                        # "探头信息列，修改探头信息"
                      }
                      frame 4, 5 {
                        w643 = T2."修改报警限值"  # 修改限值
                        # "一级限值列"
                        n312 = And(x=w646, y=w645) -> (x .and. y?=w644:bool)
                      }
                      frame 6 {
                        w647 = T2."删除设备"  # 删除设备
                        w648 = TRUE  # T
                        # "“添加”或“删除”设备"
                      }
                    }
                  }
                }
              }
            }
            n313 = case shown="真" w599 {
              tunnel: w600 -> [_ w617]
              frame False {
              }
              frame True {
                # "是否触发"
                n314 = property on="菜单项-实时列表" class="Enum (严格)"("Val(Sgnl)"=w617) -> ()  [unwired: 2 in, 2 out]
              }
            }
          }
          event "报警记录列表": Double Click {
            # "历史数据列表双击，删除记录提示"
            n315 = event-data() -> ("CtlRef"=w655:refnum<vi>, "Coords"=w663:T15, "PlatMods"=w661:T17)  [unwired: 1 in, 6 out]
            n316 = invoke class="多列列表框 (严格)" method="Point To Row Column"(reference=w655, "Point"=w663) -> ("CellPosition"=w664:T3)  [unwired: 5 in, 6 out]
            "点到行列-报警记录" <- w664
            n317 = Unbundle By Name(w661) -> ("Shift"=w660:bool, "Ctrl"=w659:bool)
            n318 = property class="MCListbox (严格)"(reference=w655) -> ("ItemNames"=w654:string[][])  [unwired: 1 in, 2 out]
            n319 = Not Or(1:w659, 2:w660) -> (0:w657:bool)
            n320 = Unbundle By Name(w664) -> ("Row"=w650:i32)  [unwired: 1 out]
            n321 = Array Size(array=w654) -> (size(s)=w653:i32[])
            n322 = Index Array(array=w653) -> (element=w652:i32)  [unwired: 1 in]
            n323 = Greater Or Equal To 0? "非标题行？"(x=w650) -> (x >= 0?=w662:bool)
            n324 = Decrement(x=w652) -> (x-1=w651:i32)
            n325 = Greater Or Equal? "有效行？"(x=w651, y=w650) -> (x >= y?=w649:bool)
            n326 = And(x=w649, y=w662) -> (x .and. y?=w656:bool)
            n327 = And(x=w656, y=w657) -> (x .and. y?=w658:bool)
            n328 = case shown="真" w658 {
              frame False {
                # "无效行"
              }
              frame True {
                # "有效行"
                n329 = property on="菜单项-报警列表" class="Enum (严格)"("Val(Sgnl)"=enum16{"刷新", "预览并生成报表", "删除记录"}."预览并生成报表" ("菜单项-报警列表")) -> ()  [unwired: 2 in, 2 out]
              }
            }
          }
          event "实时数据列表": Shortcut Menu Activation? {
            w666 = FALSE ("已启用")
            w672 = "修改报警限值" ("项名称")
            w681 = "禁用" ("项名称")
            w680 = "启用" ("项名称")
            # "“启用/禁用”始终不可用"
            # "禁用？"
            # "启用？"
            # "配置菜单项-实时列表"
            n330 = event-data() -> ("CtlRef"=w675:refnum<vi>, "MenuRef"=w674:refnum<k9>)  [unwired: 1 in, 5 out]
            n331 = property class="多列列表框 (严格)"(reference=w675) -> ("Value"=w684:i32[])  [unwired: 1 in, 2 out]
            n332 = Array Size(array=w684) -> (size(s)=w682:i32)
            n333 = Equal?(x=w682, y=1) -> (x = y?=w679:bool)
            n334 = case shown="假" w679 {
              tunnel: [w687 w689] -> _
              tunnel: [w687 w698] -> _
              tunnel: w684 -> [_ w697]
              tunnel: [w687 w688] -> w670
              frame False {
                w687 = TRUE  # T
                # "多线选择"
              }
              frame True {
                # "单项选择，根据启用状态动态修改菜单项"
                n335 = local read "探头属性数组"() -> (w695:T1)
                n336 = Index Array(array=w697) -> (element=w696:i32)  [unwired: 1 in]
                n337 = Index Array(array=w695, index=w696) -> (element=w694:T14)
                n338 = Unbundle By Name(w694) -> ("探头状态"=w692:enum16{"正常", "离线", "禁用", "一级报警", "二级报警"})
                n339 = Not Equal?(x=enum16{"正常", "离线", "禁用", "一级报警", "二级报警"}."离线" ("探头状态"), y=w692) -> (x != y?=w690:bool)
                n340 = Not Equal?(x=w692, y=enum16{"正常", "离线", "禁用", "一级报警", "二级报警"}."禁用" ("探头状态")) -> (x != y?=w689:bool)
                n341 = Not(x=w689) -> (.not. x?=w698:bool)
                n342 = And "连接？"(x=w690, y=w689) -> (x .and. y?=w688:bool)
              }
            }
            n343 = Set Menu Item Info(7:w680, 9:w666, 10:w680, 11:w674) -> (0:w677:errorcluster, 3:w678:refnum<k9>)  [unwired: 3 in]
            n344 = Set Menu Item Info(7:w681, 8:w677, 9:w666, 10:w681, 11:w678) -> (0:w667:errorcluster, 3:w668:refnum<k9>)  [unwired: 2 in]
            n345 = disable-structure shown="启用" {
              disable-tunnel: [w685 w686] -> w671
              disable-tunnel: w670 -> [w685 _]
              frame Enabled {
              }
              frame Disabled {
                w686 = TRUE  # T
              }
            }
            n346 = Set Menu Item Info(7:w672, 8:w667, 9:w671, 10:w672, 11:w668) -> ()  [unwired: 2 in, 2 out]
            n347 = local read "暂停更新？"() -> (w669:bool)
            n348 = Empty Array?(array=w684) -> (empty?=w683:bool)
            n349 = Or(x=w683, y=w669) -> (x .or. y?=w673:bool)
            n350 = event-data("Discard?"=w673) -> ()  [unwired: 1 in, 1 out]
          }
          event "报警记录列表": Shortcut Menu Activation? {
            w700 = "预览并生成报表" ("项标识符")
            # "菜单项启用状态，仅单选可 ”打开报表预览“ 项"
            n351 = event-data() -> ("CtlRef"=w708:refnum<vi>, "MenuRef"=w704:refnum<k9>)  [unwired: 1 in, 5 out]
            n352 = property class="多列列表框 (严格)"(reference=w708) -> ("Value"=w703:i32[])  [unwired: 1 in, 2 out]
            n353 = Array Size(array=w703) -> (size(s)=w702:i32)
            n354 = Equal? "单项？"(x=w702, y=1) -> (x = y?=w699:bool)
            n355 = Set Menu Item Info(7:w700, 9:w699, 10:w700, 11:w704) -> ()  [unwired: 3 in, 2 out]
            n356 = local read "暂停更新？"() -> (w705:bool)
            n357 = Empty Array?(array=w703) -> (empty?=w707:bool)
            n358 = Or(x=w707, y=w705) -> (x .or. y?=w706:bool)
            n359 = event-data("Discard?"=w706) -> ()  [unwired: 1 in, 1 out]
          }
          event "实时数据列表": Shortcut Menu Selection (User) {
            # "实时列表-菜单选择"
            n360 = event-data() -> ("ItemTag"=w711:string)  [unwired: 1 in, 7 out]
            n361 = property on="菜单项-实时列表" class="Enum (严格)"() -> ("Strings []"=w710:string[])  [unwired: 2 in, 2 out]
            n362 = for "For循环" {
              tunnel: w710 -> [w715] mode=indexing
              tunnel: w711 -> [w714]
              tunnel: [w712] -> w709
              i -> [w712]
              stop <- w713 stop-if-true
              # "寻找匹配项"
              n363 = Equal?(x=w715, y=w714) -> (x = y?=w713:bool)
            }
            n364 = property on="菜单项-实时列表" class="Enum (严格)"("Val(Sgnl)"=w709) -> ()  [unwired: 2 in, 2 out]
          }
          event "报警记录列表": Shortcut Menu Selection (User) {
            # "处理报警列表菜单事件"
            n365 = event-data() -> ("ItemTag"=w718:string)  [unwired: 1 in, 7 out]
            n366 = property on="菜单项-报警列表" class="Enum (严格)"() -> ("Strings []"=w717:string[])  [unwired: 2 in, 2 out]
            n367 = for "For循环" {
              tunnel: w717 -> [w722] mode=indexing
              tunnel: w718 -> [w721]
              tunnel: [w719] -> w716
              i -> [w719]
              stop <- w720 stop-if-true
              # "寻找匹配项"
              n368 = Equal?(x=w722, y=w721) -> (x = y?=w720:bool)
            }
            n369 = property on="菜单项-报警列表" class="Enum (严格)"("Val(Sgnl)"=w716) -> ()  [unwired: 2 in, 2 out]
          }
          event "菜单项-实时列表": Value Change {
            # "实时列表，菜单事件处理"
            n370 = event-data() -> ("CtlRef"=w726:refnum<vi>)  [unwired: 1 in, 5 out]
            n371 = local read "点到行列-实时列表"() -> (w725:T3)
            n372 = local read "暂停更新？"() -> (w724:bool)
            n373 = case shown="假" w724 {
              tunnel: w726 -> [w735 _]
              tunnel: w725 -> [w731 _]
              frame False {
                w729 = T18 {"探头信息"="", "启用？"=FALSE, "改动项"=enum."未改动", "限值"={"限值1"=1.0, "限值2"=100.0}}  # 改动项
                # "非暂停发送状态，可以产生菜单事件"
                n374 = local read "通信分支-改动项引用[]"() -> (w730:refnum<vi>[])
                n375 = property class="Enum (严格)"(reference=w735) -> ("RingText.Text"=w734:string)  [unwired: 1 in, 2 out]
                n376 = local read "在线探头索引映射"() -> (w727:i32[])
                n377 = local read "实时数据列表"() -> (w733:i32[])
                n378 = local read "探头属性数组"() -> (w732:T1)
                n379 = case shown="\"添加设备\"" w734 {
                  tunnel: w733 -> [_ w737 w758 w790 w839 _ _ w905]
                  tunnel: w732 -> [_ w736 w757 w789 w837 _ w859 w904]
                  tunnel: w731 -> [_ _ _ _ _ _ _ _]
                  tunnel: w729 -> [_ w739 w760 w788 _ _ _ _]
                  tunnel: w730 -> [_ w738 w759 w787 w838 _ _ _]
                  tunnel: "探头信息变更：\n" -> [_ _ _ w784 _ _ _ _]
                  tunnel: w727 -> [_ _ _ w783 w836 _ _ _]
                  frame "nothing", Default {
                    # "（什么也没有）"
                  }
                  frame "启用" {
                    # "启用探头"
                    n380 = disable-structure shown="禁用" {
                      disable-tunnel: w739 -> [w743 _]
                      disable-tunnel: w738 -> [w742 _]
                      disable-tunnel: w737 -> [w741 _]
                      disable-tunnel: w736 -> [w740 _]
                      frame Disabled {
                        n381 = for "For循环" {
                          tunnel: w741 -> [w748] mode=indexing
                          tunnel: w742 -> [w756]
                          tunnel: w743 -> [w753]
                          tunnel: w740 -> [w750]
                          w755 = TRUE  # T
                          # "按列表选中项索引，修改"
                          n382 = Index Array(array=w750, index=w748) -> (element=w749:T14)
                          n383 = Unbundle By Name(w749) -> ("探头地址与信息.探头信息"=w746:string)
                          n384 = Index Array(array=w756, index=w748) -> (element=w754:refnum<vi>)
                          n385 = Increment(x=w748) -> (x+1=w747:i32)
                          n386 = call "状态信息-启用"("探头号"=w747, "探头信息"=w746) -> ("Result"=w745:string)  [unwired: 12 in, 1 out]
                          n387 = Bundle By Name(cluster=w753, "改动项"=enum16{"未改动", "改动-探头信息", "改动-启用状态", "改动-限值"}."改动-启用状态", "启用？"=w755) -> (w752:T18)
                          n388 = property class="Ctl"(reference=w754, "Value"=w752) -> ()  [unwired: 1 in, 2 out]
                          n389 = call "状态栏-插入状态信息-35点监测专用.vi"("消息内容"=w745, "状态类型"=enum16{"全部", "报警", "通信", "设置"}."设置") -> ()  [unwired: 10 in]
                        }
                      }
                      frame Enabled {
                      }
                    }
                  }
                  frame "禁用" {
                    # "禁用探头"
                    n390 = disable-structure shown="禁用" {
                      disable-tunnel: w760 -> [w764 _]
                      disable-tunnel: w759 -> [w763 _]
                      disable-tunnel: w758 -> [w762 _]
                      disable-tunnel: w757 -> [w761 _]
                      frame Disabled {
                        n391 = for "For循环" {
                          tunnel: w762 -> [w770] mode=indexing
                          tunnel: w763 -> [w778]
                          tunnel: w764 -> [w775]
                          tunnel: w761 -> [w772]
                          w777 = FALSE  # F
                          # "按列表选中项索引，修改"
                          n392 = Index Array(array=w772, index=w770) -> (element=w771:T14)
                          n393 = Unbundle By Name(w771) -> ("探头地址与信息.探头信息"=w768:string)
                          n394 = Index Array(array=w778, index=w770) -> (element=w776:refnum<vi>)
                          n395 = Increment(x=w770) -> (x+1=w769:i32)
                          n396 = call "状态信息-禁用"("探头号"=w769, "探头信息"=w768) -> ("Result"=w767:string)  [unwired: 12 in, 1 out]
                          n397 = Bundle By Name(cluster=w775, "改动项"=enum16{"未改动", "改动-探头信息", "改动-启用状态", "改动-限值"}."改动-启用状态", "启用？"=w777) -> (w774:T18)
                          n398 = property class="Ctl"(reference=w776, "Value"=w774) -> (error out=w766:errorcluster)  [unwired: 1 in, 1 out]
                          n399 = call "状态栏-插入状态信息-35点监测专用.vi"("消息内容"=w767, "状态类型"=enum16{"全部", "报警", "通信", "设置"}."设置") -> ()  [unwired: 10 in]
                          n400 = call <vilib>:"Clear Errors.vi"("error in (no error)"=w766) -> ()  [unwired: 6 in, 1 out]
                        }
                      }
                      frame Enabled {
                      }
                    }
                  }
                  frame "修改探头信息" {
                    # "允许多项修改"
                    n401 = global read "全局变量-35点监测.vi" "屏幕键盘？"() -> (w782:bool)
                    n402 = case shown="真" w782 {
                      tunnel: [_ w791] -> w781
                      frame False {
                      }
                      frame True {
                        # "打开软键盘"
                        n403 = call "cmd启动屏幕键盘.vi"("软键盘开关"=enum16{"关闭", "打开"}."打开") -> ("error out"=w791:errorcluster)  [unwired: 10 in]
                      }
                    }
                    n404 = for "For循环" {
                      tunnel: w790 -> [w794] mode=indexing
                      tunnel: w789 -> [w801]
                      tunnel: w788 -> [w807]
                      tunnel: w787 -> [w798]
                      shift-right: [w802] -> w785
                      shift-left: w784 -> [w803]
                      tunnel: w783 -> [w799]
                      shift-right: [errorcluster {"status"=FALSE, "code"=0, "source"=""} ("error out")] -> w779
                      shift-left: w781 -> [_]
                      # "依次修改"
                      n405 = Increment(x=w794) -> (x+1=w806:i32)
                      n406 = Index Array(array=w801, index=w794) -> (element=w800:T14)
                      n407 = Search 1D Array(1D array=w799, element=w794) -> (index of element=w797:i32)  [unwired: 1 in]
                      n408 = Unbundle By Name(w800) -> ("探头地址与信息.探头信息"=w805:string)
                      n409 = call "构建提示"("探头地址"=w806) -> ("Result"=w811:string, "error out"=w808:errorcluster)  [unwired: 13 in]
                      n410 = Greater Or Equal To 0?(x=w797) -> (x >= 0?=w795:bool)
                      n411 = Index Array(array=w798, index=w797) -> (element=w796:refnum<vi>)
                      n412 = call "弹窗-提示修改备注-30.vi"("信息输入"=w811, "新的探头信息："=w805, "error in (no error)"=w808) -> ("新备注"=w809:string, "确定"=w810:bool)  [unwired: 14 in, 1 out]
                      n413 = case shown="真" w810 {
                        tunnel: w809 -> [_ w815]
                        tunnel: w794 -> [_ w816]
                        tunnel: w807 -> [_ w814]
                        tunnel: w806 -> [_ w824]
                        tunnel: w805 -> [_ w823]
                        tunnel: [_ w821] -> w804
                        tunnel: w801 -> [_ w818]
                        tunnel: w800 -> [_ w817]
                        tunnel: w796 -> [_ w813]
                        tunnel: w795 -> [_ w812]
                        frame False {
                          # "取消不修改"
                        }
                        frame True {
                          # "确定则修改，不经过通信分支实例\n因为被修改设备 离线时没有实例"
                          n414 = case shown="真" w812 {
                            tunnel: w818 -> [w829 _]
                            tunnel: w817 -> [w828 _]
                            tunnel: w816 -> [w826 _]
                            tunnel: w815 -> [w825 w834]
                            tunnel: w814 -> [_ w833]
                            tunnel: w813 -> [_ w831]
                            frame False {
                              # "被改项  离线，改“探头属性数组”"
                              n415 = Bundle By Name(cluster=w828, "探头地址与信息.探头信息"=w825) -> (w827:T14)
                              n416 = Replace Array Subset(array=w829, new element=w827, index=w826) -> (w830:T1)
                              n417 = local write "探头属性数组"(w830) -> ()
                            }
                            frame True {
                              # "被改项 在线，改“通信分支实例”"
                              n418 = Bundle By Name(cluster=w833, "改动项"=enum16{"未改动", "改动-探头信息", "改动-启用状态", "改动-限值"}."改动-探头信息", "探头信息"=w834) -> (w832:T18)
                              n419 = property class="Ctl"(reference=w831, "Val(Sgnl)"=w832) -> ()  [unwired: 1 in, 2 out]
                            }
                          }
                          n420 = call "构建状态信息"("探头序号"=w824, "原探头信息"=w823, "新探头信息"=w815) -> ("Result"=w822:string)  [unwired: 11 in, 1 out]
                          n421 = Concatenate Strings("L-----------------------------------" ("字符串"), w822, "\r") -> (w821:string)
                        }
                      }
                      n422 = Concatenate Strings(w803, w804) -> (w802:string)
                    }
                    n423 = call "cmd启动屏幕键盘.vi"("error in (no error)"=w779, "软键盘开关"=enum16{"关闭", "打开"}."关闭") -> ()  [unwired: 9 in, 1 out]
                    n424 = call "状态栏-插入状态信息-35点监测专用.vi"("消息内容"=w785, "状态类型"=enum16{"全部", "报警", "通信", "设置"}."设置") -> ()  [unwired: 10 in]
                  }
                  frame "修改报警限值" {
                    # "允许批量修改"
                    n425 = stacked-sequence {
                      tunnel: w839 -> [_ w841 _]
                      tunnel: w838 -> [_ w845 _]
                      tunnel: w837 -> [_ _ _]
                      tunnel: w836 -> [_ w842 _]
                      frame #0 {
                        w840 = TRUE  # T
                        # "暂停更新列表"
                        n426 = local write "暂停更新？"(w840) -> ()
                      }
                      frame #1 {
                        # "修改"
                        n427 = for {
                          tunnel: w842 -> [w849]
                          tunnel: w841 -> [w848] mode=indexing
                          tunnel: [w847] -> w844 mode=indexing if=w846
                          workers-P: _ -> [_]
                          # "选中项有效映射"
                          n428 = Search 1D Array(1D array=w849, element=w848) -> (index of element=w847:i32)  [unwired: 1 in]
                          n429 = Greater Or Equal To 0?(x=w847) -> (x >= 0?=w846:bool)
                        }
                        n430 = local read "在线探头"() -> (w843:T1)
                        n431 = call "修改-探头报警值-网络版.vi"("通信单元-改动项引用[]"=w845, "探头属性数组"=w843, "实时数据列表"=w844) -> ()  [unwired: 9 in]
                      }
                      frame #2 {
                        w850 = FALSE  # F
                        # "回复更新"
                        n432 = local write "暂停更新？"(w850) -> ()
                      }
                    }
                  }
                  frame "设备排序" {
                    # "批量编辑 探头排序，进入可拖拽模式"
                    n433 = disable-structure shown="启用" {
                      frame Enabled {
                        # "暂不开放，因为貌似这种方法不比单独设置更方便"
                        n434 = stacked-sequence {
                          frame #0 {
                            w852 = TRUE  # T
                            w851 = TRUE  # T
                            # "暂停更新，启动动态效果"
                            n435 = local write "暂停更新？"(w851) -> ()
                            n436 = local write "T:G,F:B"(w852) -> ()
                          }
                          frame #1 {
                            w855 = TRUE  # T
                            w853 = TRUE  # T
                            # "进入编辑模式"
                            n437 = property on="实时数据列表" class="多列列表框 (严格)"("Allow Drop"=w853, "Allow Item Drag"=w853) -> ()  [unwired: 2 in, 2 out]
                            n438 = property on="状态与编辑" class="Bool (严格)"("Value"=w855, "DisabledEnum"=T6."Enabled" ("禁用"), "BoolText.Text"="点此完成排序" ("布尔文本.文本")) -> ()  [unwired: 2 in, 2 out]
                          }
                          frame #2 {
                            # "状态栏提示"
                            n439 = call "状态栏-插入状态信息-35点监测专用.vi"("消息内容"="**操作提示：对当前闪烁的列表“行”拖拽排序，按菜单栏左侧按钮可结束排序。", "状态类型"=enum16{"全部", "报警", "通信", "设置"}."设置") -> ()  [unwired: 10 in]
                          }
                        }
                      }
                      frame Disabled {
                      }
                    }
                  }
                  frame "添加设备" {
                    # "添加设备：IP，Port，探头名称，都不允许空"
                    n440 = call "添加设备.vi"("探头属性数组"=w859) -> ("确认？"=w861:bool, "探头属性输出"=w860:T14)  [unwired: 9 in]
                    n441 = case shown="真" w861 {
                      tunnel: w860 -> [_ w863]
                      tunnel: w859 -> [_ w862]
                      frame False {
                        # "取消添加设备"
                      }
                      frame True {
                        # "确认添加设备"
                        n442 = disable-structure shown="启用" {
                          disable-tunnel: w863 -> [w864 w899]
                          disable-tunnel: w862 -> [_ w898]
                          frame Disabled {
                            n443 = stacked-sequence {
                              seq-local: [w868 _ _] -> [_ w879 _]
                              seq-local: [w865 _ _] -> [_ _ _]
                              seq-local: [w867 _ _] -> [_ w878 _]
                              seq-local: [w866 _ _] -> [_ w877 _]
                              tunnel: w864 -> [w869 _ w891]
                              frame #0 {
                                w876 = 128  # 重入运行
                                # "创建“通信单元”实例"
                                n444 = vi-ref "探头通信分支.vi"() -> (w870:refnum<vi>)
                                n445 = property class="VI接口类型2"(reference=w870) -> ("Name"=w875:string)  [unwired: 1 in, 2 out]
                                n446 = Open VI Reference(type specifier VI Refnum (for type only)=refnum<vi> refnum ("类型说明符VI引用句柄（仅用于类型）"), vi path=w875, options=w876) -> (vi reference=w871:refnum<vi>)  [unwired: 3 in, 1 out]
                                n447 = call-by-ref "开始异步调用"(reference=w871, "探头属性"=w869) -> (reference out=w868:refnum<vi>)  [unwired: 12 in, 1 out]
                                n448 = call "通过控件名获取控件引用.vi"("控件名数组"=string[] ["停止", "改动项", "探头属性"], "VI引用"=w868) -> ("控件引用输出"=w872:refnum<vi>[])  [unwired: 7 in, 2 out]
                                n449 = Index Array(array=w872) -> (element #1=w865:refnum<vi>, element #2=w867:refnum<vi>, element #3=w866:refnum<vi>)  [unwired: 3 in]
                              }
                              frame #1 {
                                # "添加引用"
                                n450 = local read "通信单元-探头属性引用[]"() -> (w884:refnum<vi>[])
                                n451 = local read "通信分支-改动项引用[]"() -> (w882:refnum<vi>[])
                                n452 = local read "通信分支-VI引用[]"() -> (w885:refnum<vi>[])
                                n453 = Insert Into Array(array=w885, new element=w879) -> (w880:refnum<vi>[])  [unwired: 1 in]
                                n454 = Insert Into Array(array=w882, new element=w878) -> (w881:refnum<vi>[])  [unwired: 1 in]
                                n455 = Insert Into Array(array=w884, new element=w877) -> (w883:refnum<vi>[])  [unwired: 1 in]
                                n456 = local write "通信分支-VI引用[]"(w880) -> ()
                                n457 = local write "通信分支-改动项引用[]"(w881) -> ()
                                n458 = local write "通信单元-探头属性引用[]"(w883) -> ()
                              }
                              frame #2 {
                                w887 = enum16{"全部", "报警", "通信", "设置"}."设置"  # 设置
                                # "状态栏提示"
                                n459 = Unbundle By Name(w891) -> ("探头地址与信息.探头信息"=w890:string, "探头地址与信息.网络地址.IP"=w889:string, "探头地址与信息.网络地址.port"=w888:u16)
                                n460 = call "创建文本"("探头名称"=w890, "IP"=w889, "Port"=w888) -> ("Result"=w886:string)  [unwired: 11 in, 1 out]
                                n461 = call "状态栏-插入状态信息-35点监测专用.vi"("消息内容"=w886, "状态类型"=w887) -> ()  [unwired: 10 in]
                              }
                            }
                          }
                          frame Enabled {
                            n462 = Insert Into Array(array=w898, new element=w899) -> (w896:T1)  [unwired: 1 in]
                            n463 = local read "监测数量限值"() -> (w897:cluster{"min":i32, "max":i32})
                            n464 = Array Size(array=w896) -> (size(s)=w895:i32)
                            n465 = local write "探头属性数组"(w896) -> ()
                            n466 = Unbundle By Name(w897) -> ("max"=w894:i32, "min"=w893:i32)
                            n467 = In Range and Coerce(upper limit=w894, x=w895, lower limit=w893) -> (In Range?=w892:bool)  [unwired: 1 out]
                            n468 = case shown="真" w892 {
                              frame False {
                              }
                              frame True {
                                # "超出范围，停止监测VI"
                                n469 = local read "监-停止信号"() -> (w902:refnum<vi>)
                                n470 = property class="Ctl"(reference=w902, "Val(Sgnl)"=TRUE) -> (error out=w900:errorcluster)  [unwired: 1 in, 1 out]
                                n471 = call <vilib>:"Clear Errors.vi"("error in (no error)"=w900) -> ()  [unwired: 6 in, 1 out]
                              }
                            }
                          }
                        }
                      }
                    }
                  }
                  frame "删除设备" {
                    n472 = Reverse 1D Array(array=w905) -> (reversed array=w903:i32[])
                    n473 = stacked-sequence {
                      seq-local: [w907 _ _ _ _] -> [_ w929 w950 _ _]
                      seq-local: [_ w927 _ _ _] -> [_ _ w948 w964 _]
                      seq-local: [_ w926 _ _ _] -> [_ _ _ w963 _]
                      seq-local: [_ _ w947 _ _] -> [_ _ _ _ w976]
                      tunnel: w903 -> [w908 _ _ _ _]
                      tunnel: w904 -> [w909 w928 w949 _ _]
                      frame #0 {
                        # "查看是否离线，仅能删除离线探头"
                        n474 = local read "在线探头"() -> (w906:T1)
                        n475 = for {
                          tunnel: w909 -> [w916]
                          tunnel: w908 -> [w913] mode=indexing
                          tunnel: [w913] -> w907 mode=indexing if=w914
                          tunnel: w906 -> [w912]
                          # "获取通信状态，仅选中离线设备，索引"
                          n476 = Index Array(array=w916, index=w913) -> (element=w911:T14)
                          n477 = Unbundle By Name(w911) -> ("探头地址与信息.网络地址"=w910:cluster{"IP":string, "port":u16})
                          n478 = for {
                            tunnel: w912 -> [w923] mode=indexing
                            tunnel: [w917] -> w915
                            tunnel: w910 -> [w921]
                            stop <- w917 stop-if-true
                            # "是否选中了在线设备？"
                            n479 = Unbundle By Name(w923) -> ("探头地址与信息.网络地址"=w922:cluster{"IP":string, "port":u16})
                            n480 = Equal? ("等于？")(x=w922, y=w921) -> (x = y?=w920:cluster{"IP":bool, "port":bool})
                            n481 = Unbundle By Name(w920) -> ("IP"=w919:bool, "port"=w918:bool)
                            n482 = And(x=w919, y=w918) -> (x .and. y?=w917:bool)
                          }
                          n483 = Not(x=w915) -> (.not. x?=w914:bool)
                        }
                      }
                      frame #1 {
                        # "弹窗提示"
                        n484 = for "For循环" {
                          N -> [w946]
                          tunnel: w929 -> [w937] mode=indexing
                          tunnel: w928 -> [w944]
                          shift-right: [w932] -> w926
                          shift-left: "" -> [w934]
                          i -> [w945]
                          # "构建-删除清单"
                          n485 = Decrement(x=w946) -> (x-1=w942:i32)
                          n486 = Equal?(x=w942, y=w945) -> (x = y?=w941:bool)
                          n487 = Index Array(array=w944, index=w937) -> (element=w943:T14)
                          n488 = Unbundle By Name(w943) -> ("探头地址与信息.探头信息"=w936:string)
                          n489 = Increment(x=w937) -> (x+1=w931:i32)
                          n490 = Select(t="", s=w941, f="\r\n") -> (s? t:f=w938:string)
                          n491 = call "构建探头信息2"("探头号"=w931, "探头信息"=w936) -> ("Result"=w935:string)  [unwired: 12 in, 1 out]
                          n492 = Concatenate Strings(w935, w938) -> (w933:string)
                          n493 = Concatenate Strings(w934, w933) -> (w932:string)
                        }
                        n494 = Concatenate Strings("删除设备？\n（在线设备不可删除）\n" ("字符串"), w926) -> (w924:string)
                        n495 = call "将删除以下设备"("Message"=w924) -> ("删除"=w927:bool)  [unwired: 9 in, 1 out]
                      }
                      frame #2 {
                        # "探头属性数组中  删除选中的离线条目"
                        n496 = case shown="真" w948 {
                          tunnel: w950 -> [_ w958]
                          tunnel: w949 -> [w952 w956]
                          tunnel: [w951 w953] -> w947
                          frame False {
                            # "取消删除"
                            n497 = Array Size(array=w952) -> (size(s)=w951:i32)
                          }
                          frame True {
                            # "确认删除"
                            n498 = Sort 1D Array(array=w958) -> (sorted array=w957:i32[])
                            n499 = Reverse 1D Array(array=w957) -> (reversed array=w955:i32[])
                            n500 = for {
                              shift-right: [w959] -> w954
                              shift-left: w956 -> [w961]
                              tunnel: w955 -> [w960] mode=indexing
                              # "索引从大到小  删除"
                              n501 = Delete From Array(array=w961, index=w960) -> (array with subset deleted=w959:T1)  [unwired: 1 in, 1 out]
                            }
                            n502 = local write "探头属性数组"(w954) -> ()
                            n503 = Array Size(array=w954) -> (size(s)=w953:i32)
                          }
                        }
                      }
                      frame #3 {
                        # "状态提示，回到顶部（删除超过一页时需要回顶）"
                        n504 = property on="实时数据列表" class="MCListbox (严格)"("TopLeft"=T4 {"Row"=0, "Column"=0} ("左上可见单元格")) -> ()  [unwired: 2 in, 2 out]
                        n505 = case shown="真" w964 {
                          tunnel: w963 -> [_ w969]
                          frame False {
                            # "取消删除"
                          }
                          frame True {
                            w970 = enum16{"全部", "报警", "通信", "设置"}."设置"  # 设置
                            w975 = TRUE  # T
                            # "删除"
                            n506 = Empty String/Path?(string/path=w969) -> (empty?=w967:bool)
                            n507 = Search and Replace String(replace all?=w975, input string=w969, search string="\r\n", replace string="，") -> (result string=w972:string)  [unwired: 4 in, 3 out]
                            n508 = Concatenate Strings("已移除设备：", w972) -> (w968:string)
                            n509 = Select(t="在线设备不可删除", s=w967, f=w968) -> (s? t:f=w965:string)
                            n510 = call "状态栏-插入状态信息-35点监测专用.vi"("消息内容"=w965, "状态类型"=w970) -> ()  [unwired: 10 in]
                          }
                        }
                      }
                      frame #4 {
                        # "判断设备数量是否在监测窗口显示范围内"
                        n511 = local read "监测数量限值"() -> (w980:cluster{"min":i32, "max":i32})
                        n512 = Unbundle By Name(w980) -> ("max"=w979:i32, "min"=w978:i32)
                        n513 = In Range and Coerce(upper limit=w979, x=w976, lower limit=w978) -> (In Range?=w977:bool)  [unwired: 1 out]
                        n514 = case shown="真" w977 {
                          frame False {
                          }
                          frame True {
                            # "超出范围，停止监测VI"
                            n515 = local read "监-停止信号"() -> (w983:refnum<vi>)
                            n516 = property class="Ctl"(reference=w983, "Val(Sgnl)"=TRUE) -> (error out=w981:errorcluster)  [unwired: 1 in, 1 out]
                            n517 = call <vilib>:"Clear Errors.vi"("error in (no error)"=w981) -> ()  [unwired: 6 in, 1 out]
                          }
                        }
                      }
                    }
                  }
                }
              }
              frame True {
                # "不产生菜单事件"
              }
            }
          }
          event "菜单项-报警列表": Value Change {
            # "报警列表，菜单事件处理"
            n518 = event-data() -> ("CtlRef"=w986:refnum<vi>)  [unwired: 1 in, 5 out]
            n519 = local read "点到行列-报警记录"() -> (w985:T3)
            n520 = local read "暂停更新？"() -> (w984:bool)
            n521 = case shown="假" w984 {
              tunnel: w986 -> [w992 _]
              tunnel: w985 -> [w990 _]
              frame False {
                # "非暂停，可执行"
                n522 = local read "报警记录列表"() -> (w987:i32[])
                n523 = local read "报警记录缓存数据文件"() -> (w989:string[])
                n524 = property class="Enum (严格)"(reference=w992) -> ("RingText.Text"=w991:string)  [unwired: 1 in, 2 out]
                n525 = Unbundle By Name(w990) -> ()  [unwired: 1 out]
                n526 = for "For循环" {
                  tunnel: w989 -> [w995]
                  tunnel: [w994] -> w988 mode=indexing
                  tunnel: w987 -> [w993] mode=indexing
                  workers-P: _ -> [_]
                  n527 = Index Array(array=w995, index=w993) -> (element=w994:string)
                }
                n528 = case shown="\"删除记录\"" w991 {
                  tunnel: w988 -> [_ _ w1015 w1051 _]
                  tunnel: w987 -> [_ _ w1012 _ w1069]
                  frame "假", Default {
                  }
                  frame "刷新" {
                    # "刷新报警记录清单"
                    n529 = call "读取-缓存数据文件夹至报警记录列表-网络版.vi"() -> ("文件名"=→"报警记录缓存数据文件":string[], "新记录文件名"=w996:string[], "新记录列表"=w997:string[][], "报警记录列表"=w1001:string[][])  [unwired: 8 in]
                    n530 = Array Size(array=w1001) -> (size(s)=w1000:i32[])
                    n531 = for {
                      workers-P: _ -> [_]
                      tunnel: w997 -> [w1007] mode=indexing
                      tunnel: w996 -> [w1006] mode=indexing
                      tunnel: [w1005] -> w998 mode=indexing
                      # "数组到簇绑定"
                      n532 = Bundle("新记录列表"=w1007, "字符串"=w1006) -> (w1005:cluster{"新记录列表":string[], "字符串":string})  [unwired: 1 in]
                    }
                    n533 = Index Array(array=w1000) -> (element=w999:i32)  [unwired: 1 in]
                    n534 = local write "报警记录数"(w999) -> ()
                    n535 = property on="新记录簇" class="Arr (严格)"("Val(Sgnl)"=w998) -> ()  [unwired: 2 in, 2 out]
                    n536 = property on="报警记录列表" class="MCListbox (严格)"("ItemNames"=w1001, "Value"=i32[] [] ("报警记录列表"), "TopLeft"=T4 {"Row"=0, "Column"=0} ("左上可见单元格")) -> ()  [unwired: 2 in, 2 out]
                  }
                  frame "预览并生成报表" {
                    # "避免空选"
                    # "获得文件路径，预览并生成报表"
                    n537 = property on="报警记录列表" class="MCListbox (严格)"() -> ("ItemNames"=w1013:string[][])  [unwired: 2 in, 2 out]
                    n538 = Index Array(array=w1012) -> (element=w1011:i32)  [unwired: 1 in]
                    n539 = Increment(x=w1011) -> (x+1=w1009:i32)
                    n540 = Array Size(array=w1013) -> (size(s)=w1014:i32[])
                    n541 = Index Array(array=w1014) -> (element=w1010:i32)  [unwired: 1 in]
                    n542 = Greater Or Equal? "有效行？"(x=w1010, y=w1009) -> (x >= y?=w1008:bool)
                    n543 = case shown="真" w1008 {
                      tunnel: w1015 -> [_ w1016]
                      frame False {
                      }
                      frame True {
                        # "有效行"
                        n544 = call "路径查找创建-报警记录清单-网络版.vi"() -> ("缓存数据文件夹"=w1017:path)  [unwired: 1 in, 10 out]
                        n545 = vi-ref "预览报表-服务器版.vi"() -> (w1018:refnum<vi>)
                        n546 = disable-structure shown="启用" {
                          disable-tunnel: w1018 -> [w1021 w1047]
                          disable-tunnel: w1017 -> [w1020 w1048]
                          disable-tunnel: w1016 -> [w1019 w1050]
                          frame Disabled {
                            # "预分配重入"
                            n547 = for "For循环" {
                              tunnel: w1021 -> [w1028]
                              tunnel: w1020 -> [w1024]
                              tunnel: w1019 -> [w1022] mode=indexing
                              # "打开多个窗口？"
                              n548 = property class="VI"(reference=w1028) -> ("Name"=w1027:string)  [unwired: 1 in, 2 out]
                              n549 = Build Path(base path=w1024, name or relative path=w1022) -> (appended path=w1023:path)
                              n550 = Open VI Reference(type specifier VI Refnum (for type only)=refnum<vi> refnum ("类型说明符VI引用句柄（仅用于类型）"), vi path=w1027, options=128 ("选项")) -> (vi reference=w1025:refnum<vi>)  [unwired: 3 in, 1 out]
                              n551 = call-by-ref "开始异步调用"(reference=w1025, "缓存数据路径"=w1023) -> ()  [unwired: 12 in, 2 out]
                            }
                          }
                          frame Enabled {
                            # "共享副本重入"
                            n552 = Index Array(array=w1050) -> (element=w1049:string)  [unwired: 1 in]
                            n553 = Build Path(base path=w1048, name or relative path=w1049) -> (appended path=w1040:path)
                            n554 = invoke class="VI" method="FP.Open"(reference=w1047, "Activate"=TRUE ("激活？"), "State"=T5."Hidden" ("状态")) -> (reference out=w1044:refnum<vi>, error out=w1031:errorcluster)  [unwired: 2 in, 3 out]
                            n555 = call "通过控件名获取控件引用.vi"("控件名数组"=string[] ["缓存数据路径"], "VI引用"=w1044) -> ("控件引用输出"=w1042:refnum<vi>[], "VI引用o"=w1039:refnum<vi>)  [unwired: 7 in, 1 out]
                            n556 = Index Array(array=w1042) -> (element=w1041:refnum<vi>)  [unwired: 1 in]
                            n557 = property class="Ctl"(reference=w1041, error in=w1031, "Val(Sgnl)"=w1040) -> (error out=w1030:errorcluster)  [unwired: 1 out]
                            n558 = invoke class="VI" method="Run VI"(reference=w1039, error in=w1030, "Wait until done"=FALSE ("结束前等待"), "Auto Dispose Ref"=TRUE ("自动销毁引用")) -> (reference out=w1036:refnum<vi>, error out=w1035:errorcluster)  [unwired: 1 in, 3 out]
                            n559 = invoke class="VI" method="FP.Open"(reference=w1036, error in=w1035, "Activate"=TRUE ("激活？"), "State"=T5."Standard" ("状态")) -> (error out=w1032:errorcluster)  [unwired: 1 in, 4 out]
                            n560 = call <vilib>:"Clear Errors.vi"("error in (no error)"=w1032) -> ()  [unwired: 6 in, 1 out]
                          }
                        }
                      }
                    }
                  }
                  frame "删除记录" {
                    # "删除缓存的xml文件，然后刷新"
                    n561 = stacked-sequence {
                      seq-local: [w1052 _ _ _] -> [_ _ w1059 _]
                      seq-local: [_ w1058 _ _] -> [_ _ w1060 _]
                      tunnel: w1051 -> [w1053 _ _ _]
                      frame #0 {
                        # "删除缓存数据xml文件"
                        n562 = call "路径查找创建-报警记录清单-网络版.vi"() -> ("缓存数据文件夹"=w1054:path)  [unwired: 1 in, 10 out]
                        n563 = for "For循环" {
                          tunnel: w1054 -> [w1057]
                          tunnel: w1053 -> [w1056] mode=indexing
                          tunnel: [w1055] -> w1052 mode=indexing
                          workers-P: _ -> [_]
                          n564 = Build Path(base path=w1057, name or relative path=w1056) -> (appended path=w1055:path)
                        }
                      }
                      frame #1 {
                        # "弹窗确认"
                        n565 = call "显示对话框信息"() -> ("确定"=w1058:bool)  [unwired: 10 in, 1 out]
                      }
                      frame #2 {
                        # "删除操作"
                        n566 = case shown="真" w1060 {
                          tunnel: w1059 -> [_ w1061]
                          frame False {
                          }
                          frame True {
                            n567 = for "For循环" {
                              tunnel: w1061 -> [w1063] mode=indexing
                              n568 = Delete(path (use dialog)=w1063) -> (error out=w1062:errorcluster)  [unwired: 4 in, 2 out]
                              n569 = call <vilib>:"Clear Errors.vi"("error in (no error)"=w1062) -> ()  [unwired: 6 in, 1 out]
                            }
                          }
                        }
                      }
                      frame #3 {
                        # "刷新列表"
                        n570 = call "读取-缓存数据文件夹至报警记录列表-网络版.vi"() -> ("文件名"=w1065:string[], "报警记录列表"=w1066:string[][])  [unwired: 8 in, 2 out]
                        n571 = local write "报警记录缓存数据文件"(w1065) -> ()
                        n572 = property on="报警记录列表" class="MCListbox (严格)"("ItemNames"=w1066, "Value"=i32[] [] ("报警记录列表")) -> ()  [unwired: 2 in, 2 out]
                      }
                    }
                  }
                  frame "复制选中项至剪贴板" {
                    # "复制选中行到剪贴板"
                    n573 = property on="报警记录列表" class="MCListbox (严格)"() -> ("ItemNames"=w1073:string[][])  [unwired: 2 in, 2 out]
                    n574 = for {
                      tunnel: w1073 -> [w1085] mode=indexing
                      tunnel: [w1086] -> w1074 mode=indexing
                      tunnel: [w1085] -> w1076
                      n575 = To Variant(anything=w1085) -> (Variant=w1086:variant)
                    }
                    n576 = call "重排数组.vi"("新索引顺序"=w1069, "原数组"=w1074) -> ("排序后数组"=w1075:variant[])  [unwired: 9 in]
                    n577 = call "状态栏-插入状态信息-35点监测专用.vi"("消息内容"="已复制 报警记录列表选中项 至剪贴板", "状态类型"=enum16{"全部", "报警", "通信", "设置"}."设置") -> ()  [unwired: 10 in]
                    n578 = for {
                      tunnel: w1075 -> [w1084] mode=indexing
                      tunnel: w1076 -> [w1083]
                      tunnel: [w1082] -> w1077 mode=indexing
                      n579 = Variant To Data(type=w1083, Variant=w1084) -> (data=w1082:string[])  [unwired: 1 in, 1 out]
                    }
                    n580 = Array To Spreadsheet String(array=w1077, 3:"%s" ("格式字符串")) -> (spreadsheet string=w1080:string)  [unwired: 1 in]
                    n581 = Array To Spreadsheet String(array=string[] ["报警时间", "探头信息", "最大值(μSv/h)", "报警等级", "网络地址"] ("ItemNames"), 3:"%s" ("格式字符串")) -> (spreadsheet string=w1067:string)  [unwired: 1 in]
                    n582 = control-ref of="本应用程序"() -> (w1079:refnum<vi>)
                    n583 = Concatenate Strings(w1067, w1080) -> (w1081:string)
                    n584 = invoke class="App" method="Clipboard.Write"(reference=w1079, "Param 0"=w1081) -> ()  [unwired: 2 in, 4 out]
                  }
                }
              }
              frame True {
                # "暂停发送，不执行"
              }
            }
          }
          event "状态与编辑": Value Change {
            n585 = event-data() -> ("OldVal"=w1089:bool, "NewVal"=w1088:bool)  [unwired: 1 in, 4 out]
            n586 = Not Equal?(x=w1089, y=w1088) -> (x != y?=w1087:bool)
            n587 = case "条件结构" shown="真" w1087 {
              tunnel: w1088 -> [_ w1090]
              frame False {
                # "值未改变"
              }
              frame True {
                # "值有变化"
                n588 = case shown="假" w1090 {
                  frame False {
                    # "点击  结束修改"
                    n589 = stacked-sequence {
                      seq-local: [w1091 _ _ _] -> [_ w1097 _ _]
                      seq-local: [_ w1096 _ _] -> [_ _ w1108 _]
                      frame #0 {
                        w1094 = 0  # 编号列
                        # "获得排序后的编号顺序"
                        n590 = property on="实时数据列表" class="MCListbox (严格)"() -> ("ItemNames"=w1095:string[][])  [unwired: 2 in, 2 out]
                        n591 = Index Array "探头序号咧"(array=w1095, index (col)=w1094) -> (element=w1093:string[])  [unwired: 1 in]
                        n592 = Decimal String To Number(string=w1093) -> (number=w1092:i32[])  [unwired: 2 in, 1 out]
                        n593 = Decrement(x=w1092) -> (x-1=w1091:i32[])
                      }
                      frame #1 {
                        # "改变“探头属性数”的顺序，改变“在线探头索引映射”的顺序"
                        n594 = local read "在线探头索引映射"() -> (w1098:i32[])
                        n595 = local read "探头属性数组"() -> (w1100:T1)
                        n596 = for {
                          tunnel: w1097 -> [w1106] mode=indexing
                          tunnel: w1100 -> [w1107]
                          tunnel: [w1105] -> w1099 mode=indexing
                          workers-P: _ -> [_]
                          # "重新排序"
                          n597 = Index Array(array=w1107, index=w1106) -> (element=w1105:T14)
                        }
                        n598 = for {
                          tunnel: w1098 -> [w1103]
                          tunnel: w1097 -> [w1104] mode=indexing
                          tunnel: [w1101] -> w1096 mode=indexing if=w1102
                          workers-P: _ -> [_]
                          # "重排索引"
                          n599 = Search 1D Array(1D array=w1103, element=w1104) -> (index of element=w1101:i32)  [unwired: 1 in]
                          n600 = Greater Or Equal To 0?(x=w1101) -> (x >= 0?=w1102:bool)
                        }
                        n601 = local write "探头属性数组"(w1099) -> ()
                        n602 = local write "在线探头索引映射"(w1096) -> ()
                      }
                      frame #2 {
                        # "注意：不要出现空的行"
                        # "更改受影响的项"
                        n603 = local read "通信单元-探头属性引用[]"() -> (w1113:refnum<vi>[])
                        n604 = local read "通信分支-改动项引用[]"() -> (w1112:refnum<vi>[])
                        n605 = local read "通信分支-VI引用[]"() -> (w1114:refnum<vi>[])
                        n606 = stacked-sequence "依次重排" {
                          tunnel: w1114 -> [w1120 _ _]
                          tunnel: w1113 -> [_ w1127 _]
                          tunnel: w1112 -> [_ _ w1139]
                          tunnel: w1108 -> [w1118 w1130 w1141]
                          tunnel: [w1116 _ _] -> w1111
                          tunnel: [_ w1128 _] -> w1110
                          tunnel: [_ _ w1138] -> w1109
                          frame #0 {
                            n607 = for "For循环" {
                              workers-P: _ -> [_]
                              tunnel: w1120 -> [w1124] mode=indexing
                              tunnel: [w1125] -> w1119 mode=indexing
                              tunnel: [w1124] -> w1115
                              n608 = To Variant(anything=w1124) -> (Variant=w1125:variant)
                            }
                            n609 = call "重排数组.vi"("新索引顺序"=w1118, "原数组"=w1119) -> ("排序后数组"=w1117:variant[])  [unwired: 9 in]
                            n610 = for "For循环" {
                              workers-P: _ -> [_]
                              tunnel: w1117 -> [w1123] mode=indexing
                              tunnel: [w1122] -> w1116 mode=indexing
                              tunnel: w1115 -> [w1121]
                              n611 = Variant To Data(type=w1121, Variant=w1123) -> (data=w1122:refnum<vi>)  [unwired: 1 in, 1 out]
                            }
                          }
                          frame #1 {
                            n612 = for "For循环" {
                              workers-P: _ -> [_]
                              tunnel: w1127 -> [w1135] mode=indexing
                              tunnel: [w1136] -> w1131 mode=indexing
                              tunnel: [w1135] -> w1126
                              n613 = To Variant(anything=w1135) -> (Variant=w1136:variant)
                            }
                            n614 = call "重排数组.vi"("新索引顺序"=w1130, "原数组"=w1131) -> ("排序后数组"=w1129:variant[])  [unwired: 9 in]
                            n615 = for "For循环" {
                              workers-P: _ -> [_]
                              tunnel: w1129 -> [w1134] mode=indexing
                              tunnel: [w1133] -> w1128 mode=indexing
                              tunnel: w1126 -> [w1132]
                              n616 = Variant To Data(type=w1132, Variant=w1134) -> (data=w1133:refnum<vi>)  [unwired: 1 in, 1 out]
                            }
                          }
                          frame #2 {
                            n617 = for "For循环" {
                              workers-P: _ -> [_]
                              tunnel: w1139 -> [w1146] mode=indexing
                              tunnel: [w1147] -> w1142 mode=indexing
                              tunnel: [w1146] -> w1137
                              n618 = To Variant(anything=w1146) -> (Variant=w1147:variant)
                            }
                            n619 = call "重排数组.vi"("新索引顺序"=w1141, "原数组"=w1142) -> ("排序后数组"=w1140:variant[])  [unwired: 9 in]
                            n620 = for "For循环" {
                              workers-P: _ -> [_]
                              tunnel: w1140 -> [w1145] mode=indexing
                              tunnel: [w1144] -> w1138 mode=indexing
                              tunnel: w1137 -> [w1143]
                              n621 = Variant To Data(type=w1143, Variant=w1145) -> (data=w1144:refnum<vi>)  [unwired: 1 in, 1 out]
                            }
                          }
                        }
                        n622 = local write "通信分支-VI引用[]"(w1111) -> ()
                        n623 = local write "通信单元-探头属性引用[]"(w1110) -> ()
                        n624 = local write "通信分支-改动项引用[]"(w1109) -> ()
                      }
                      frame #3 {
                        w1150 = FALSE  # F
                        # "更改标志，使在状态机中检测到更改，状态栏提示"
                        n625 = local write "暂停更新？"(w1150) -> ()
                        n626 = property on="状态与编辑" class="Bool (严格)"("DisabledEnum"=T6."Disabled" ("禁用")) -> ()  [unwired: 2 in, 2 out]
                        n627 = call "状态栏-插入状态信息-35点监测专用.vi"("消息内容"="探头排序完成", "状态类型"=enum16{"全部", "报警", "通信", "设置"}."设置") -> ()  [unwired: 10 in]
                      }
                    }
                  }
                  frame True {
                    # "不执行"
                  }
                }
              }
            }
          }
          event "新记录？": Value Change {
            # "刷新列表"
            n628 = event-data() -> ()  [unwired: 1 in, 6 out]
            n629 = property on="菜单项-报警列表" class="Enum (严格)"("Val(Sgnl)"=enum16{"刷新", "预览并生成报表", "删除记录"}."刷新" ("菜单项-报警列表")) -> ()  [unwired: 2 in, 2 out]
          }
          event "设置": Value Change {
            (unwired) FALSE ("值(信号)")
            # "设置"
            n630 = event-data() -> ()  [unwired: 1 in, 6 out]
          }
          event Panel Resize {
            # "允许全屏窗口"
            # "允许纵向调整"
            n631 = event-data() -> ("VIRef"=w1154:refnum<vi>, "NewBnds"=w1153:T13)  [unwired: 1 in, 6 out]
            n632 = disable-structure shown="禁用" {
              disable-tunnel: w1154 -> [w1159 _]
              disable-tunnel: w1153 -> [w1158 _]
              frame Disabled {
                n633 = Bundle By Name(cluster=w1158, "Left"="Left", "Right"="Right") -> (w1155:T13)
                n634 = property class="VI"(reference=w1159, "Front Panel.PanelBounds"=w1155) -> ()  [unwired: 1 in, 2 out]
              }
              frame Enabled {
              }
            }
          }
        }
        "最终事件" <- w262
      }
      n635 = local read "定时循环结构名称"() -> (w84:string)
      n636 = node-c288(w84, i64 2000 ("偏移量")) -> (w86:T7)  [unwired: 8 in]
      n637 = timed-loop {
        timing: w86 -> [_]
        timing-out: [_] -> w85
        stop <- _ stop-if-true
        # "周期性，从“通信分支”收集探头信息"
        n638 = node-c288() -> ()  [unwired: 1 in, 3 out]
        n639 = stacked-sequence {
          seq-local: [w126 _ _ _] -> [_ w151 _ _]
          seq-local: [_ w148 _ _] -> [_ _ w178 _]
          frame #0 {
            w127 = T14 {"探头地址与信息"={"网络地址"={"IP"="", "port"=0}, "探头信息"=""}, "测量值"={"时间"=timestamp(3554955153.6246996 s since 1904-01-01), "数值"=0.0}, "限值"={"限值1"=0.0, "限值2"=0.0}, "探头状态"=enum."正常"}  # 探头属性
            # "收集探头属性，并以“信号”形式赋值，供监测窗口事件捕捉"
            n640 = for "For循环" {
              tunnel: "通信单元-探头属性引用[]" -> [w136] mode=indexing
              tunnel: w127 -> [w134]
              tunnel: [w131] -> w126 mode=indexing
              tunnel: [w129] -> w125 mode=indexing
              i -> [w130]
              # "从“通信单元”获取属性值"
              n641 = property class="Ctl"(reference=w136) -> (error out=w133:errorcluster, "Value"=w135:variant)  [unwired: 1 in, 1 out]
              n642 = Variant To Data(error in=w133, type=w134, Variant=w135) -> (data=w132:T14, error out=w129:errorcluster)
              n643 = case shown="错误" w129 {
                tunnel: w132 -> [w139 w144]
                tunnel: [w139 w145] -> w131
                tunnel: w130 -> [w137 w142]
                frame No Error {
                  # "通信分支实例运行正常"
                  n644 = Unbundle By Name(w139) -> ("探头状态"=w138:enum16{"正常", "离线", "禁用", "一级报警", "二级报警"})
                  n645 = case shown="\"离线\"" w138 {
                    tunnel: w137 -> [_ w141]
                    frame "正常", Default {
                    }
                    frame "离线" {
                      # "离线释放"
                      n646 = local read "连接断开-事件"() -> (w140:refnum<user-event>)
                      n647 = Generate User Event(user event=w140, event data cluster=w141) -> ()  [unwired: 2 in, 2 out]
                    }
                  }
                }
                frame Error {
                  # "数据引用异常，产生断开连接事件"
                  n648 = local read "连接断开-事件"() -> (w143:refnum<user-event>)
                  n649 = Bundle By Name(cluster=w144, "探头状态"=enum16{"正常", "离线", "禁用", "一级报警", "二级报警"}."离线") -> (w145:T14)
                  n650 = Generate User Event(user event=w143, event data cluster=w142) -> ()  [unwired: 2 in, 2 out]
                }
              }
            }
            "在线探头" <- w126
            "数组" <- w125
          }
          frame #1 {
            # "整理探头属性数组"
            n651 = for {
              tunnel: w151 -> [w155] mode=indexing
              shift-right: [w153] -> w148
              shift-left: "探头属性数组" -> [w156]
              tunnel: [w152] -> w149 mode=indexing
              # "以“在线探头”为索引"
              n652 = for {
                tunnel: w156 -> [w170] mode=indexing
                tunnel: w155 -> [w171]
                tunnel: [w169] -> w157
                tunnel: [w168] -> w154
                i -> [w168]
                stop <- w169 stop-if-true
                # "匹配并替换"
                n653 = Unbundle By Name(w171) -> ("探头地址与信息.网络地址"=w173:cluster{"IP":string, "port":u16})
                n654 = Unbundle By Name(w170) -> ("探头地址与信息.网络地址"=w172:cluster{"IP":string, "port":u16})
                n655 = Equal?(x=w172, y=w173) -> (x = y?=w176:cluster{"IP":bool, "port":bool})
                n656 = Unbundle By Name(w176) -> ("IP"=w175:bool, "port"=w174:bool)
                n657 = And "匹配？"(x=w175, y=w174) -> (x .and. y?=w169:bool)
              }
              n658 = case shown="假" w157 {
                tunnel: w156 -> [w162 w167]
                tunnel: w155 -> [w161 w166]
                tunnel: w154 -> [w159 w164]
                tunnel: [w160 w165] -> w153
                tunnel: [w158 w164] -> w152
                frame False {
                  n659 = Insert Into Array(array=w162, new element=w161) -> (w160:T1)  [unwired: 1 in]
                  n660 = Increment(x=w159) -> (x+1=w158:i32)
                  n661 = Unbundle By Name(w161) -> ("探头地址与信息.网络地址.IP"=w163:string)
                  n662 = call "显示对话框信息5"("Message"=w163) -> ()  [unwired: 9 in, 2 out]
                }
                frame True {
                  n663 = Replace Array Subset(array=w167, new element=w166, index=w164) -> (w165:T1)
                }
              }
            }
            "在线探头索引映射" <- w149
            n664 = Array Size(array=w148) -> (size(s)=w147:i32)
            n665 = property on="探头属性数组" class="Arr (严格)"("Val(Sgnl)"=w148) -> ()  [unwired: 2 in, 2 out]
            n666 = local write "所有探头数"(w147) -> ()
          }
          frame #2 {
            # "更新实时列表"
            n667 = case shown="假" "暂停更新？" {
              tunnel: w178 -> [w186 _]
              tunnel: "监测模式？" -> [w185 _]
              frame False {
                # "整理与更新"
                n668 = case shown="假" w185 {
                  tunnel: w186 -> [w188 w193]
                  tunnel: [w187 w190] -> w184
                  frame False {
                    # "管理模式，刷新列表"
                    n669 = control-ref of="实时数据列表"() -> (w189:refnum<vi>)
                    n670 = call "整合-测量信息至列表框-网络版.vi"("MCListbox引用句柄"=w189, "探头属性数组"=w188) -> ("测量状态"=w187:enum16{"正常", "一级报警", "二级报警"})  [unwired: 9 in]
                  }
                  frame True {
                    # "监测模式，不刷新，仅判断检测状态"
                    n671 = for {
                      workers-P: _ -> [_]
                      tunnel: w193 -> [w198] mode=indexing
                      tunnel: [w197] -> w192 mode=indexing
                      n672 = Unbundle By Name(w198) -> ("探头状态"=w197:enum16{"正常", "离线", "禁用", "一级报警", "二级报警"})
                    }
                    n673 = Array Max & Min(array=w192) -> (max value=w191:enum16{"正常", "离线", "禁用", "一级报警", "二级报警"})  [unwired: 3 out]
                    n674 = case shown="\"一级报警\"" w191 {
                      tunnel: [enum16{"正常", "一级报警", "二级报警"}."正常" enum16{"正常", "一级报警", "二级报警"}."一级报警" enum16{"正常", "一级报警", "二级报警"}."二级报警"] -> w190
                      frame "正常", Default {
                      }
                      frame "一级报警" {
                      }
                      frame "二级报警" {
                      }
                    }
                  }
                }
                n675 = Get Date/Time String(want seconds? (F)=TRUE ("需要秒？(F)")) -> (time string=w183:string)  [unwired: 2 in, 1 out]
                n676 = Concatenate Strings("更新时间  " ("字符串"), w183) -> (w182:string)
                n677 = property on="状态与编辑" class="Bool (严格)"("BoolText.Text"=w182) -> ()  [unwired: 2 in, 2 out]
                n678 = local write "测量状态"(w184) -> ()
              }
              frame True {
                # "设置过程中（排序中），不更新"
              }
            }
          }
          frame #3 {
            # "更新时间"
          }
        }
        n679 = node-c288() -> ()  [unwired: 1 in, 1 out]
      }
      n680 = node-c288(w85) -> ()  [unwired: 1 out]
      n681 = while {
        stop <- w207 stop-if-true
        # "列表动态效果"
        n682 = local read "暂停更新？"() -> (w206:bool)
        n683 = case shown="假" w206 {
          selector: w206 -> [_ w225]
          frame False {
            n684 = local write "等待时间（毫秒）"(u32 1000 ("等待时间（毫秒）")) -> ()
            n685 = case shown="真" "回复背景色锁" {
              selector: "回复背景色锁" -> [_ w220]
              frame False {
              }
              frame True {
                w218 = -2 ("Column")
                n686 = Not(x=w220) -> (.not. x?=w219:bool)
                n687 = local write "回复背景色锁"(w219) -> ()
                n688 = Bundle("Column"=w218, "Column"=w218) -> (w215:cluster{"Column":i32, "Column":i32})  [unwired: 1 in]
                n689 = property on="实时数据列表" class="MCListbox (严格)"("ActiveCell"=w215, "CellBG"=u32 16777226) -> (error out=w212:errorcluster)  [unwired: 2 in, 1 out]
                n690 = Bundle("Column"=-1, "Column"=-2) -> (w213:cluster{"Column":i32, "Column":i32})  [unwired: 1 in]
                n691 = property on="实时数据列表" class="MCListbox (严格)"(error in=w212, "ActiveCell"=w213, "CellBG"=u32 13816530) -> ()  [unwired: 1 in, 2 out]
              }
            }
          }
          frame True {
            w223 = -2 ("Column")
            w226 = u8 20 ("B动态范围")
            # "处于编辑模式的列表，背景色渐变"
            n692 = local write "回复背景色锁"(w225) -> ()
            n693 = feedback #2(0.0 ("y")) -> (w234:dbl)
            n694 = Greater Or Equal?(x=w234, y=1.0) -> (x >= y?=w229:bool)
            n695 = feedback #3(0.05 ("y")) -> (w232:dbl)
            n696 = Add(x=w234, y=w232) -> (x+y=w237:dbl)
            n697 = feedback-in #2(w237) -> ()
            n698 = case shown="假" w229 {
              tunnel: [w246 -0.05 ("y")] -> w231
              tunnel: w234 -> [w249 _]
              tunnel: w232 -> [w247 _]
              frame False {
                n699 = Less Or Equal?(x=w249, y=-1.0) -> (x <= y?=w245:bool)
                n700 = case shown="真" w245 {
                  tunnel: w247 -> [w250 _]
                  tunnel: [w250 0.05 ("y")] -> w246
                  frame False {
                  }
                  frame True {
                    # "-1"
                    n701 = Wait (ms)(milliseconds to wait=u32 0 ("等待时间（毫秒）")) -> ()  [unwired: 1 out]
                  }
                }
              }
              frame True {
                # "1"
                n702 = Wait (ms)(milliseconds to wait=u32 0 ("等待时间（毫秒）")) -> ()  [unwired: 1 out]
              }
            }
            n703 = Multiply(x=3.141592653589793, y=w237) -> (x*y=w239:dbl)
            n704 = Cosine(x=w239) -> (cos(x)=w240:dbl)
            n705 = Multiply(x=w240, y=w226) -> (x*y=w230:dbl)
            n706 = Add(x=w230, y=w226) -> (x+y=w228:dbl)
            n707 = Absolute Value(x=w228) -> (abs(x)=w241:dbl)
            n708 = case shown="假" "T:G,F:B" {
              tunnel: w241 -> [w256 w260]
              tunnel: [w257 w259] -> w243
              tunnel: [w255 w258] -> w242
              frame False {
                w257 = u8 255 ("G")
                # "B"
                n709 = Subtract(x=w257, y=w256) -> (x-y=w255:dbl)
              }
              frame True {
                w258 = u8 255 ("G")
                # "G"
                n710 = Subtract(x=w258, y=w260) -> (x-y=w259:dbl)
              }
            }
            n711 = feedback-in #3(w231) -> ()
            n712 = Bundle("Column"=w223, "Column"=w223) -> (w221:cluster{"Column":i32, "Column":i32})  [unwired: 1 in]
            n713 = call <vilib>:"RGB to Color.vi"("B"=w243, "G"=w242, "R"=u8 125 ("R常量")) -> ("Color"=w222:u32)
            n714 = local write "等待时间（毫秒）"(u32 0 ("等待时间（毫秒）")) -> ()
            n715 = property on="实时数据列表" class="多列列表框 (严格)"("ActiveCell"=w221, "CellBG"=w222) -> ()  [unwired: 2 in, 2 out]
          }
        }
        n716 = Wait (ms)(milliseconds to wait="等待时间（毫秒）") -> ()  [unwired: 1 out]
        n717 = local read "停止"() -> (w207:bool)
      }
      n718 = TCP Create Listener(10:u16 60000 ("端口")) -> (0:w78:errorcluster, 2:w75:u16, 3:w77:refnum<k5>)  [unwired: 4 in]
      n719 = local read "蜂鸣音效"() -> (w83:waveform(dbl)[])
      n720 = while {
        tunnel: "设备列表提示" -> [w93]
        stop <- w92 stop-if-true
        # "设备列表循环提示"
        n721 = for {
          tunnel: w93 -> [w94] mode=indexing
          tunnel: [w95] -> w92
          stop <- w95 stop-if-true
          n722 = local read "停止"() -> (w95:bool)
          n723 = Wait (ms)(milliseconds to wait=u32 5000 ("等待时间（毫秒）")) -> ()  [unwired: 1 out]
          "设备列表操作提示" <- w94
        }
      }
      n724 = case shown="错误" w78 {
        tunnel: w77 -> [w97 w103]
        tunnel: [w97 w101] -> w76
        tunnel: w75 -> [_ w102]
        frame No Error {
        }
        frame Error {
          n725 = TCP Close Connection(connection ID=w103, abort (F)=TRUE ("中止(F)")) -> (error out=w100:errorcluster)  [unwired: 1 in, 1 out]
          n726 = TCP Create Listener(8:w100, 10:w102) -> (0:w99:errorcluster, 3:w101:refnum<k5>)  [unwired: 3 in, 1 out]
          n727 = call <vilib>:"Clear Errors.vi"("error in (no error)"=w99) -> ()  [unwired: 6 in, 1 out]
        }
      }
      n728 = local read "新连接-事件"() -> (w81:refnum<user-event>)
      n729 = while {
        tunnel: w83 -> [w116]
        stop <- w123 stop-if-true
        w118 = enum16{"正常", "一级报警", "二级报警"}."二级报警"  # 二级报警
        # "报警声音播放"
        n730 = case shown="\"正常\"" "测量状态" {
          tunnel: w116 -> [_ w124]
          frame "正常" {
          }
          frame "一级报警", Default {
            n731 = call "播放波形"("Data"=w124) -> ()  [unwired: 18 in, 1 out]
          }
        }
        n732 = Equal?(x="测量状态", y=w118) -> (x = y?=w119:bool)
        n733 = Select(t=u32 0 ("等待时间（毫秒）"), s=w119, f=u32 500 ("等待时间（毫秒）")) -> (s? t:f=w122:u32)
        n734 = Wait (ms)(milliseconds to wait=w122) -> ()  [unwired: 1 out]
        n735 = local read "停止"() -> (w123:bool)
      }
      n736 = while {
        tunnel: w76 -> [w113]
        tunnel: w81 -> [w111]
        tunnel: w80 -> [w109]
        stop <- w112 stop-if-true
        # "等待侦听，有新连接时产生事件"
        n737 = TCP Wait On Listener(9:2000 ("超时毫秒（一直等待:-1）"), 11:w113) -> (0:w104:errorcluster, 1:w107:u16, 2:w108:string, 4:w106:refnum<k5>)  [unwired: 2 in, 1 out]
        n738 = Bundle By Name(cluster=w109, "IP地址"=w108, "端口"=w107, "连接ID"=w106) -> (w110:T11)
        n739 = case shown="错误" w104 {
          tunnel: w111 -> [w115 _]
          tunnel: w110 -> [w114 _]
          frame No Error {
            n740 = Generate User Event(user event=w115, event data cluster=w114) -> ()  [unwired: 2 in, 2 out]
          }
          frame Error {
          }
        }
        n741 = local read "停止"() -> (w112:bool)
      }
      n742 = while {
        tunnel: "报警列表提示" -> [w88]
        stop <- w87 stop-if-true
        # "设备列表循环提示"
        n743 = for {
          tunnel: w88 -> [w89] mode=indexing
          tunnel: [w90] -> w87
          stop <- w90 stop-if-true
          n744 = local read "停止"() -> (w90:bool)
          n745 = Wait (ms)(milliseconds to wait=u32 5000 ("等待时间（毫秒）")) -> ()  [unwired: 1 out]
          "报警列表操作提示" <- w89
        }
      }
    }
  }
